vi "V(I)_K2636B_PK.vi"() -> ()   [LabVIEW 2016]
uses:
  Application/Labview Drivers/Keithley 2600 Series/Public/Configure/Source/Configure Source (Limit).vi
  Application/Labview Drivers/Keithley 2600 Series/Public/Configure/Source/Configure Source (Range).vi
  Labview Drivers/Keithley 2600 Series/Public/Data/Read Measurement (Current and Voltage).vi
  Application/Labview Drivers/Keithley 2600 Series/Keithley 2600 Series.lvlib
panel:
  in  "4-point sense":bool=TRUE
  out "Resistance (ohm)":dbl=6608698.625453053 format="%#_13g"
  out "R vs V":cluster{dbl, "Field Reading":dbl}[](graph)=[{3.33548e-05, "Field Reading"=75621777.7515791}, {3.15428e-05, "Field Reading"=1576.9586497552782}, {3.19242e-05, "Field Reading"=797.9912862417107}, {3.13759e-05, "Field Reading"=522.8758932380546}, {3.35217e-05, "Field Reading"=418.980923086153}, {3.21865e-05, "Field Reading"=321.8392528597712}, {3.17812e-05, "Field Reading"=264.76169847630314}, {3.32117e-05, "Field Reading"=237.178992772874}, {3.36409e-05, "Field Reading"=210.20570114597783}, {3.27587e-05, "Field Reading"=181.93819631888212}, {3.33786e-05, "Field Reading"=166.85295529073022}, {3.28064e-05, "Field Reading"=149.08205184134948}, {3.19719e-05, "Field Reading"=133.19072177832584}, {3.27826e-05, "Field Reading"=126.06025648420527}, {3.20911e-05, "Field Reading"=114.59142718391132}, {3.31402e-05, "Field Reading"=110.44487620850427}, {3.37124e-05, "Field Reading"=105.33413320335445}, {3.19719e-05, "Field Reading"=94.01619676064786}, {3.04937e-05, "Field Reading"=84.68449203801315}, {3.25918e-05, "Field Reading"=85.75074458792453}, {3.10421e-05, "Field Reading"=77.58915025132285}, {3.25918e-05, "Field Reading"=77.58529983788686}, {3.25441e-05, "Field Reading"=73.94974595758991}, {3.20196e-05, "Field Reading"=69.59678138034617}, {3.03268e-05, "Field Reading"=63.16977862207446}, {3.09229e-05, "Field Reading"=61.83293874874027}, {2.90155e-05, "Field Reading"=55.7893826068565}, {3.00884e-05, "Field Reading"=55.70935537385946}, {2.91348e-05, "Field Reading"=52.01797565038539}, {3.13044e-05, "Field Reading"=53.963613295592836}, {3.03507e-05, "Field Reading"=50.576660617604276}, {3.16858e-05, "Field Reading"=51.09747542754856}, {2.99692e-05, "Field Reading"=46.81992516735797}, {3.11136e-05, "Field Reading"=47.133891118311915}, {2.86102e-05, "Field Reading"=42.06646189857952}, {2.87533e-05, "Field Reading"=41.0698650349161}, {2.96354e-05, "Field Reading"=41.153761765498245}, {2.9397e-05, "Field Reading"=39.719717718017975}, {2.84672e-05, "Field Reading"=37.45112588078662}, {3.11852e-05, "Field Reading"=39.97569554828587}, {3.11375e-05, "Field Reading"=38.91623214633878}, {3.05891e-05, "Field Reading"=37.29918631973379}, {2.89917e-05, "Field Reading"=34.50932732778487}, {2.94447e-05, "Field Reading"=34.2332067232401}, {2.97546e-05, "Field Reading"=33.807857890329494}, {3.3474e-05, "Field Reading"=37.18854014371481}, {3.24249e-05, "Field Reading"=35.240319614653934}, {3.03745e-05, "Field Reading"=32.30941386833285}, {3.14236e-05, "Field Reading"=32.72933689544373}, {3.10183e-05, "Field Reading"=31.647871099788087}, {3.16858e-05, "Field Reading"=31.682314945356012}, {3.33786e-05, "Field Reading"=32.719947457676966}, {3.29733e-05, "Field Reading"=31.702352681017988}, {3.20911e-05, "Field Reading"=30.27290908061808}, {3.47137e-05, "Field Reading"=32.141124402799896}, {3.34263e-05, "Field Reading"=30.38284992319369}, {3.31163e-05, "Field Reading"=29.563901585487788}, {3.33548e-05, "Field Reading"=29.25526036504609}, {3.34263e-05, "Field Reading"=28.813043590693987}, {2.95877e-05, "Field Reading"=25.07283466235054}, {3.04461e-05, "Field Reading"=25.370904303189892}, {3.06368e-05, "Field Reading"=25.108220850851097}, {3.06606e-05, "Field Reading"=24.723299600854734}, {3.10898e-05, "Field Reading"=24.672290514320178}, {3.18766e-05, "Field Reading"=24.901259256944662}, {3.20196e-05, "Field Reading"=24.628756470705873}, {3.20911e-05, "Field Reading"=24.307204047779553}, {3.09706e-05, "Field Reading"=23.108938964333678}, {3.23057e-05, "Field Reading"=23.751396894482998}, {3.05414e-05, "Field Reading"=22.1292042836234}, {3.20196e-05, "Field Reading"=22.869509320762806}, {3.19719e-05, "Field Reading"=22.514471219525934}, {3.25918e-05, "Field Reading"=22.630051381752537}, {3.37362e-05, "Field Reading"=23.103979619090666}, {3.12805e-05, "Field Reading"=21.133188303967138}, {3.00407e-05, "Field Reading"=20.025531290830067}, {2.97308e-05, "Field Reading"=19.558450101966976}, {3.01838e-05, "Field Reading"=19.596816080610814}, {3.09944e-05, "Field Reading"=19.865658248942445}, {3.03745e-05, "Field Reading"=19.222298866577646}, {3.02315e-05, "Field Reading"=18.892916289097897}, {3.01838e-05, "Field Reading"=18.63048027010178}, {3.02315e-05, "Field Reading"=18.43282990567591}, {3.21388e-05, "Field Reading"=19.358273953295065}, {3.12805e-05, "Field Reading"=18.617239716936776}, {2.99454e-05, "Field Reading"=17.613179858484738}, {3.31879e-05, "Field Reading"=19.293608115571317}, {3.3021e-05, "Field Reading"=18.976168447184982}, {3.1352e-05, "Field Reading"=17.81090400904407}, {3.12805e-05, "Field Reading"=17.571044190919153}, {3.20435e-05, "Field Reading"=17.79967004216128}, {3.23057e-05, "Field Reading"=17.748531746685785}, {3.35693e-05, "Field Reading"=18.242499334300632}, {3.11613e-05, "Field Reading"=16.752036126118863}, {3.07322e-05, "Field Reading"=16.344393683953005}, {3.22819e-05, "Field Reading"=16.988148990138193}, {3.32356e-05, "Field Reading"=17.308134962999222}, {3.12805e-05, "Field Reading"=16.122306978661992}, {3.08514e-05, "Field Reading"=15.738904193449649}, {3.02553e-05, "Field Reading"=15.277831079511598}, {2.97546e-05, "Field Reading"=14.87499437587174}, {3.06845e-05, "Field Reading"=15.188391593161276}, {3.32356e-05, "Field Reading"=16.290124152669062}, {3.25203e-05, "Field Reading"=15.785020871760022}, {3.14951e-05, "Field Reading"=15.140637544046882}, {3.14236e-05, "Field Reading"=14.96162416439713}, {3.09467e-05, "Field Reading"=14.595847639889824}, {3.08752e-05, "Field Reading"=14.425978273566171}, {2.91109e-05, "Field Reading"=13.47589597355825}, {3.0756e-05, "Field Reading"=14.106962663975784}, {3.11613e-05, "Field Reading"=14.162038594035467}, {3.13282e-05, "Field Reading"=14.109767961374938}, {3.24011e-05, "Field Reading"=14.46277524092648}, {3.09706e-05, "Field Reading"=13.702228947112278}, {3.32594e-05, "Field Reading"=14.585984747152699}, {3.12567e-05, "Field Reading"=13.588569788976706}, {3.10898e-05, "Field Reading"=13.398696753951974}, {3.07798e-05, "Field Reading"=13.151849731235632}, {3.32117e-05, "Field Reading"=14.07096555522603}, {3.18289e-05, "Field Reading"=13.371970406718567}, {3.18289e-05, "Field Reading"=13.260605101114049}, {3.46661e-05, "Field Reading"=14.322526534979898}, {3.24726e-05, "Field Reading"=13.306588426202905}, {3.2711e-05, "Field Reading"=13.295479025000915}, {3.23772e-05, "Field Reading"=13.053796128678501}, {3.49998e-05, "Field Reading"=13.998408171917434}, {3.3164e-05, "Field Reading"=13.159064216106405}, {3.22104e-05, "Field Reading"=12.679462753310554}, {3.3164e-05, "Field Reading"=12.953017775052437}, {3.53336e-05, "Field Reading"=13.693548449604894}, {3.56197e-05, "Field Reading"=13.698462082783712}, {3.41654e-05, "Field Reading"=13.039084355190194}, {3.438e-05, "Field Reading"=13.020754431146795}, {3.28064e-05, "Field Reading"=12.331564149212888}, {3.47137e-05, "Field Reading"=12.951230067827217}, {3.28302e-05, "Field Reading"=12.158027471123473}, {5.20706e-05, "Field Reading"=19.141773212854652}, {5.3215e-05, "Field Reading"=19.41997357876375}, {5.37634e-05, "Field Reading"=19.47695228158646}, {5.20945e-05, "Field Reading"=18.736804623911553}, {5.32627e-05, "Field Reading"=19.020287039649183}, {5.1713e-05, "Field Reading"=18.33599262489806}, {5.22375e-05, "Field Reading"=18.391672651992057}, {5.36203e-05, "Field Reading"=18.745734862257024}, {5.35727e-05, "Field Reading"=18.599242458434162}, {5.24282e-05, "Field Reading"=18.076508007654247}, {5.28336e-05, "Field Reading"=18.091654025401237}, {5.27859e-05, "Field Reading"=17.952616918739306}, {5.31435e-05, "Field Reading"=17.952308243194853}, {5.19037e-05, "Field Reading"=17.41489454506412}, {5.29528e-05, "Field Reading"=17.648697831607997}, {5.46932e-05, "Field Reading"=18.10817253572422}, {5.49078e-05, "Field Reading"=18.059815875250386}, {5.23329e-05, "Field Reading"=17.100634253616487}, {5.56707e-05, "Field Reading"=18.072262169488226}, {5.28812e-05, "Field Reading"=17.056140780926455}, {5.53131e-05, "Field Reading"=17.726341899570244}, {5.43594e-05, "Field Reading"=17.30987112983502}, {5.45979e-05, "Field Reading"=17.27590298542883}, {5.47171e-05, "Field Reading"=17.2049039090406}, {5.50985e-05, "Field Reading"=17.215806477818816}, {5.63622e-05, "Field Reading"=17.50139732458919}, {5.61714e-05, "Field Reading"=17.334658268552435}, {5.70059e-05, "Field Reading"=17.484434329740704}, {5.66244e-05, "Field Reading"=17.261694636243085}, {5.7292e-05, "Field Reading"=17.358687221252666}, {5.6839e-05, "Field Reading"=17.117808978274095}, {5.6076e-05, "Field Reading"=16.78701009447857}, {5.76735e-05, "Field Reading"=17.162688965599333}, {5.94378e-05, "Field Reading"=17.583223138295512}, {5.65767e-05, "Field Reading"=16.638493096298912}, {5.73397e-05, "Field Reading"=16.76364136027692}, {5.84126e-05, "Field Reading"=16.978185993111367}, {5.8651e-05, "Field Reading"=16.949098664323984}, {5.5933e-05, "Field Reading"=16.07099245195195}, {5.68867e-05, "Field Reading"=16.251578400059422}, {5.94139e-05, "Field Reading"=16.87650368838606}, {5.85318e-05, "Field Reading"=16.532118435583776}, {5.99623e-05, "Field Reading"=16.84121389150248}, {6.00338e-05, "Field Reading"=16.76720393919166}, {6.00576e-05, "Field Reading"=16.680813242973002}, {6.03437e-05, "Field Reading"=16.66782676908714}, {6.06775e-05, "Field Reading"=16.667353385523967}, {5.86271e-05, "Field Reading"=16.01627659836032}, {6.02484e-05, "Field Reading"=16.369757123410867}, {6.00576e-05, "Field Reading"=16.229853747121965}, {6.08444e-05, "Field Reading"=16.354175066255962}, {6.02961e-05, "Field Reading"=16.119581344989374}, {6.001e-05, "Field Reading"=15.957899439439228}, {6.31094e-05, "Field Reading"=16.69344450058061}, {6.26802e-05, "Field Reading"=16.49274958097288}, {6.08444e-05, "Field Reading"=15.925935620317974}, {6.19412e-05, "Field Reading"=16.12867275624668}, {6.21319e-05, "Field Reading"=16.09392889151371}, {6.39439e-05, "Field Reading"=16.47809325506244}, {6.33001e-05, "Field Reading"=16.228631054320964}, {6.20842e-05, "Field Reading"=15.835867036689383}, {6.41823e-05, "Field Reading"=16.28810488168834}, {6.37531e-05, "Field Reading"=16.096910048528247}, {6.51598e-05, "Field Reading"=16.369546921907776}, {6.55174e-05, "Field Reading"=16.37718002364687}, {6.50883e-05, "Field Reading"=16.188985034311397}, {6.44922e-05, "Field Reading"=15.961479919514714}, {6.49452e-05, "Field Reading"=15.994581881318572}, {6.64234e-05, "Field Reading"=16.277931078425127}, {6.43253e-05, "Field Reading"=15.687069720255673}, {6.5732e-05, "Field Reading"=15.95247167205842}, {6.71148e-05, "Field Reading"=16.209503291904763}, {6.58512e-05, "Field Reading"=15.82794127544202}, {6.46591e-05, "Field Reading"=15.466464143902789}, {6.61135e-05, "Field Reading"=15.739173493121173}, {6.44922e-05, "Field Reading"=15.280556516464719}, {6.61612e-05, "Field Reading"=15.602216719726448}, {6.61135e-05, "Field Reading"=15.517888871415597}, {6.53028e-05, "Field Reading"=15.256095167786489}, {6.53744e-05, "Field Reading"=15.201298429514159}, {6.59227e-05, "Field Reading"=15.258012327191341}, {6.62088e-05, "Field Reading"=15.253726529201705}, {6.58035e-05, "Field Reading"=15.090849881550009}, {6.51598e-05, "Field Reading"=14.875138399022934}, {6.6185e-05, "Field Reading"=15.040028723421178}, {6.44922e-05, "Field Reading"=14.589180079401885}, {6.62088e-05, "Field Reading"=14.910112081215532}, {6.67334e-05, "Field Reading"=14.960901419565433}, {6.73532e-05, "Field Reading"=15.032518692110257}, {6.75201e-05, "Field Reading"=15.002933033512129}, {6.7687e-05, "Field Reading"=14.972979310314317}, {6.74486e-05, "Field Reading"=14.85458938155614}, {6.63996e-05, "Field Reading"=14.559559702228897}, {6.4683e-05, "Field Reading"=14.12129164092365}, {6.57082e-05, "Field Reading"=14.282807775659656}, {6.5732e-05, "Field Reading"=14.225734963121992}, {6.73771e-05, "Field Reading"=14.519080547947565}, {6.92368e-05, "Field Reading"=14.855929021252857}, {6.73771e-05, "Field Reading"=14.395247526444766}, {6.82592e-05, "Field Reading"=14.521689182001914}, {6.88076e-05, "Field Reading"=14.575935839072327}, {6.62565e-05, "Field Reading"=13.97642487538471}, {6.82831e-05, "Field Reading"=14.343501604853211}, {6.65903e-05, "Field Reading"=13.929509760444471}, {6.88076e-05, "Field Reading"=14.333423601708155}, {6.85453e-05, "Field Reading"=14.21965953456724}, {6.48737e-05, "Field Reading"=13.401995620377638}, {6.90699e-05, "Field Reading"=14.210188475061669}, {7.12872e-05, "Field Reading"=14.606356647597815}, {6.96421e-05, "Field Reading"=14.21113634647681}, {7.20501e-05, "Field Reading"=14.64284117467737}, {7.27654e-05, "Field Reading"=14.727959794601093}, {7.08103e-05, "Field Reading"=14.27454340200782}, {7.32422e-05, "Field Reading"=14.705585906833958}, {7.10487e-05, "Field Reading"=14.208233927203715}, {7.09057e-05, "Field Reading"=14.179608602270953}, {7.0262e-05, "Field Reading"=14.107220659482751}, {7.00235e-05, "Field Reading"=14.11596201258318}, {7.04288e-05, "Field Reading"=14.25499530425208}, {7.01189e-05, "Field Reading"=14.250331774551826}, {7.08103e-05, "Field Reading"=14.449489239961311}, {6.99759e-05, "Field Reading"=14.337707840304883}, {7.02143e-05, "Field Reading"=14.445633143301533}, {7.15733e-05, "Field Reading"=14.786069466738558}, {7.06196e-05, "Field Reading"=14.65000155587134}, {7.11679e-05, "Field Reading"=14.825101551921675}, {6.81162e-05, "Field Reading"=14.248700978136268}, {6.71864e-05, "Field Reading"=14.113159193790635}, {6.73532e-05, "Field Reading"=14.207797358129174}, {6.7234e-05, "Field Reading"=14.242711186525412}, {6.69956e-05, "Field Reading"=14.252957682955111}, {6.69718e-05, "Field Reading"=14.308715540466917}, {6.87599e-05, "Field Reading"=14.753697012350553}, {6.73294e-05, "Field Reading"=14.50889547813195}, {6.65903e-05, "Field Reading"=14.41164440039043}, {6.28948e-05, "Field Reading"=13.67144518471019}, {6.51121e-05, "Field Reading"=14.21512592566718}, {6.77824e-05, "Field Reading"=14.86289910558249}, {6.72102e-05, "Field Reading"=14.802215590622282}, {6.58989e-05, "Field Reading"=14.577532086590658}, {6.60658e-05, "Field Reading"=14.679853525433067}, {6.79493e-05, "Field Reading"=15.165629575402637}, {6.61612e-05, "Field Reading"=14.832686918506896}, {6.77347e-05, "Field Reading"=15.25377658472431}, {6.49214e-05, "Field Reading"=14.686338515969805}, {6.53744e-05, "Field Reading"=14.85589366832024}, {6.54936e-05, "Field Reading"=14.951374747742237}, {6.3777e-05, "Field Reading"=14.62620916141875}, {6.48737e-05, "Field Reading"=14.946238540987496}, {6.44922e-05, "Field Reading"=14.9270568847515}, {6.34193e-05, "Field Reading"=14.746856782768637}, {6.45399e-05, "Field Reading"=15.078006728343146}, {6.3014e-05, "Field Reading"=14.79056055506265}, {6.42538e-05, "Field Reading"=15.15262567092094}, {6.6185e-05, "Field Reading"=15.681865569793011}, {6.60658e-05, "Field Reading"=15.728005104129963}, {6.51598e-05, "Field Reading"=15.586455338305578}, {6.46353e-05, "Field Reading"=15.535800558118071}, {6.57082e-05, "Field Reading"=15.869897571025232}, {6.36101e-05, "Field Reading"=15.43762104231081}, {6.30617e-05, "Field Reading"=15.379064453272658}, {6.22272e-05, "Field Reading"=15.249821101232197}, {6.17981e-05, "Field Reading"=15.21974490135184}, {6.36339e-05, "Field Reading"=15.749289060817786}, {6.23465e-05, "Field Reading"=15.507266563361993}, {6.19888e-05, "Field Reading"=15.495340559132904}, {6.07967e-05, "Field Reading"=15.273633965582212}, {6.16312e-05, "Field Reading"=15.56131234629621}, {6.22749e-05, "Field Reading"=15.804207694650287}, {6.32763e-05, "Field Reading"=16.140101621246597}, {6.21557e-05, "Field Reading"=15.935356839781667}, {6.32048e-05, "Field Reading"=16.287714017708968}, {6.53744e-05, "Field Reading"=16.933960187019984}, {6.43969e-05, "Field Reading"=16.76823568316924}, {6.08206e-05, "Field Reading"=15.919872684155147}, {6.02484e-05, "Field Reading"=15.853006493984907}, {6.33001e-05, "Field Reading"=16.74393198747249}, {6.1655e-05, "Field Reading"=16.39542614014094}, {6.02484e-05, "Field Reading"=16.106958390811972}, {6.1655e-05, "Field Reading"=16.572187324447167}, {6.13689e-05, "Field Reading"=16.584306646272584}, {5.96762e-05, "Field Reading"=16.214420014998208}, {6.10828e-05, "Field Reading"=16.687192320090915}, {6.04391e-05, "Field Reading"=16.601913478680068}, {6.29902e-05, "Field Reading"=17.398925518250998}, {6.03914e-05, "Field Reading"=16.773571751949095}, {5.93424e-05, "Field Reading"=16.57414493271739}, {6.05345e-05, "Field Reading"=17.00192391411198}, {5.87702e-05, "Field Reading"=16.599453747927548}, {5.83649e-05, "Field Reading"=16.57848840512197}, {6.07014e-05, "Field Reading"=17.341374365068937}, {5.79834e-05, "Field Reading"=16.660173085542876}, {6.0606e-05, "Field Reading"=17.51410959972951}, {5.97239e-05, "Field Reading"=17.359327994884392}, {5.9557e-05, "Field Reading"=17.41193461717249}, {5.98431e-05, "Field Reading"=17.59915184952093}, {5.81503e-05, "Field Reading"=17.202449450500687}, {5.89848e-05, "Field Reading"=17.552910367813354}, {5.88655e-05, "Field Reading"=17.62218523419211}, {5.87702e-05, "Field Reading"=17.699415141275608}, {5.79834e-05, "Field Reading"=17.56822513157217}, {5.3525e-05, "Field Reading"=16.316906174359975}, {5.47409e-05, "Field Reading"=16.7897815278634}, {5.61237e-05, "Field Reading"=17.31993790909175}, {5.73635e-05, "Field Reading"=17.812372881882233}, {5.7888e-05, "Field Reading"=18.087399936259164}, {5.66244e-05, "Field Reading"=17.804623434119836}, {5.72443e-05, "Field Reading"=18.11327859256095}, {5.68151e-05, "Field Reading"=18.091906660382882}, {5.86271e-05, "Field Reading"=18.788388630908315}, {5.83887e-05, "Field Reading"=18.832573756374156}, {5.54085e-05, "Field Reading"=17.98720312682604}, {5.68628e-05, "Field Reading"=18.58079273273862}, {5.68151e-05, "Field Reading"=18.687087628357354}, {5.65052e-05, "Field Reading"=18.708162961246217}, {5.56231e-05, "Field Reading"=18.538623312302736}, {5.50032e-05, "Field Reading"=18.454786725405395}, {5.42879e-05, "Field Reading"=18.338895907791883}, {5.49793e-05, "Field Reading"=18.698597757364066}, {5.19753e-05, "Field Reading"=17.79787077399317}, {5.30243e-05, "Field Reading"=18.28209796092872}, {5.31197e-05, "Field Reading"=18.442099050462616}, {5.33104e-05, "Field Reading"=18.637523685664142}, {5.48124e-05, "Field Reading"=19.298306146950814}, {5.23329e-05, "Field Reading"=18.555791937027976}, {5.50509e-05, "Field Reading"=19.658929400421382}, {5.13792e-05, "Field Reading"=18.479533005074938}, {5.10931e-05, "Field Reading"=18.50951140607962}, {5.09977e-05, "Field Reading"=18.610669138469625}, {5.0211e-05, "Field Reading"=18.458162087447523}, {5.12838e-05, "Field Reading"=18.99203045610085}, {5.13792e-05, "Field Reading"=19.169054441260744}, {5.25713e-05, "Field Reading"=19.76112075900073}, {5.08785e-05, "Field Reading"=19.26938546724335}, {5.095e-05, "Field Reading"=19.445006316287625}, {5.03063e-05, "Field Reading"=19.34671666185944}, {4.94957e-05, "Field Reading"=19.1822237035372}, {5.04017e-05, "Field Reading"=19.68578023754936}, {4.99964e-05, "Field Reading"=19.680910110811503}, {4.89235e-05, "Field Reading"=19.412469595787652}, {5.04017e-05, "Field Reading"=20.15874476050299}, {5.10216e-05, "Field Reading"=20.57115210160266}, {5.28336e-05, "Field Reading"=21.474803476055374}, {5.06401e-05, "Field Reading"=20.751672956902667}, {4.96149e-05, "Field Reading"=20.49931414027897}, {4.9758e-05, "Field Reading"=20.730945179111565}, {4.8399e-05, "Field Reading"=20.333920116292262}, {4.91858e-05, "Field Reading"=20.839498012897103}, {4.92811e-05, "Field Reading"=21.057959372035583}, {5.00441e-05, "Field Reading"=21.568036754026433}, {5.03302e-05, "Field Reading"=21.88117348358375}, {4.67062e-05, "Field Reading"=20.483558315571575}, {4.73261e-05, "Field Reading"=20.938899212459074}, {4.62055e-05, "Field Reading"=20.625153442696128}, {4.76599e-05, "Field Reading"=21.4657160358153}, {4.59194e-05, "Field Reading"=20.86951384123146}, {4.51803e-05, "Field Reading"=20.723387274328488}, {4.64678e-05, "Field Reading"=21.510978200991584}, {4.673e-05, "Field Reading"=21.834203960340528}, {4.52995e-05, "Field Reading"=21.365370738080305}, {4.673e-05, "Field Reading"=22.249626236751638}, {4.49896e-05, "Field Reading"=21.62795169602338}, {4.52757e-05, "Field Reading"=21.976574862390663}, {4.60148e-05, "Field Reading"=22.55406332712479}, {4.68969e-05, "Field Reading"=23.213758897545816}, {4.84943e-05, "Field Reading"=24.243998280223572}, {4.60863e-05, "Field Reading"=23.27250049235213}, {4.55618e-05, "Field Reading"=23.24380028262855}, {4.59909e-05, "Field Reading"=23.704205751984333}, {4.56095e-05, "Field Reading"=23.752102612707855}, {3.34024e-05, "Field Reading"=17.577712640835248}, {3.438e-05, "Field Reading"=18.284413574501805}, {3.49998e-05, "Field Reading"=18.815579388758973}, {3.31879e-05, "Field Reading"=18.0351378669478}, {3.29494e-05, "Field Reading"=18.10197724438389}, {3.37124e-05, "Field Reading"=18.726510206915705}, {3.44992e-05, "Field Reading"=19.378742430880884}, {3.40462e-05, "Field Reading"=19.34135478446611}, {3.38316e-05, "Field Reading"=19.441772261011984}, {3.53336e-05, "Field Reading"=20.54064109569929}, {3.1209e-05, "Field Reading"=18.356075755793434}, {3.32594e-05, "Field Reading"=19.79455193634205}, {3.05176e-05, "Field Reading"=18.38132811323596}, {3.03984e-05, "Field Reading"=18.53436659736237}, {3.16143e-05, "Field Reading"=19.51331366425124}, {3.10659e-05, "Field Reading"=19.41424607539246}, {3.24965e-05, "Field Reading"=20.564801923807117}, {3.15666e-05, "Field Reading"=20.23227642432749}, {3.24488e-05, "Field Reading"=21.06722934588541}, {3.19719e-05, "Field Reading"=21.032622639151114}, {3.26633e-05, "Field Reading"=21.77364628398872}, {3.19958e-05, "Field Reading"=21.616446870608584}, {3.34263e-05, "Field Reading"=22.89159019312423}, {3.2258e-05, "Field Reading"=22.398122496024886}, {3.29494e-05, "Field Reading"=23.202659023850938}, {3.09467e-05, "Field Reading"=22.103206913791873}, {3.32117e-05, "Field Reading"=24.064182359632788}, {3.47137e-05, "Field Reading"=25.521776849782377}, {3.54528e-05, "Field Reading"=26.45356255456316}, {3.25203e-05, "Field Reading"=24.63229891761284}, {3.37124e-05, "Field Reading"=25.93101962956126}, {3.00646e-05, "Field Reading"=23.48595042613525}, {3.00884e-05, "Field Reading"=23.877597987477284}, {3.34024e-05, "Field Reading"=26.934378376634893}, {3.08275e-05, "Field Reading"=25.26471504204298}, {3.39746e-05, "Field Reading"=28.31122295923469}, {3.14474e-05, "Field Reading"=26.64875812451804}, {3.22819e-05, "Field Reading"=27.82706514149764}, {3.22819e-05, "Field Reading"=28.313978985036925}, {3.08514e-05, "Field Reading"=27.541958291672618}, {3.20435e-05, "Field Reading"=29.125953261768633}, {3.16858e-05, "Field Reading"=29.338160404436955}, {3.16858e-05, "Field Reading"=29.89057223176047}, {3.31163e-05, "Field Reading"=31.839840783009166}, {3.18766e-05, "Field Reading"=31.246973484291523}, {3.08514e-05, "Field Reading"=30.847698276206852}, {3.22342e-05, "Field Reading"=32.88804726772973}, {3.33548e-05, "Field Reading"=34.74042172031476}, {3.13759e-05, "Field Reading"=33.37417896556309}, {3.25918e-05, "Field Reading"=35.42136489163878}, {3.07798e-05, "Field Reading"=34.19483852332441}, {3.3474e-05, "Field Reading"=38.03332034272482}, {3.31402e-05, "Field Reading"=38.529292083754775}, {3.25441e-05, "Field Reading"=38.73735005154013}, {3.39746e-05, "Field Reading"=41.426679705504355}, {3.42607e-05, "Field Reading"=42.819023956167015}, {3.19719e-05, "Field Reading"=40.98352039953033}, {3.1352e-05, "Field Reading"=41.24563067584581}, {3.17335e-05, "Field Reading"=42.875691772233985}, {3.07798e-05, "Field Reading"=42.74164879967117}, {3.14951e-05, "Field Reading"=44.98458145689879}, {3.40462e-05, "Field Reading"=50.057487995153956}, {3.27826e-05, "Field Reading"=49.660899612045526}, {3.39985e-05, "Field Reading"=53.112614646293444}, {3.46422e-05, "Field Reading"=55.86298312606429}, {3.2568e-05, "Field Reading"=54.26959832698733}, {3.45469e-05, "Field Reading"=59.550478515086326}, {3.15905e-05, "Field Reading"=56.40012568869909}, {3.15666e-05, "Field Reading"=58.443462773225306}, {3.2115e-05, "Field Reading"=61.746553613658655}, {3.16381e-05, "Field Reading"=63.26114384776423}, {3.10898e-05, "Field Reading"=64.75571172379605}, {3.14951e-05, "Field Reading"=68.45287644615615}, {3.11613e-05, "Field Reading"=70.80440077799794}, {3.31163e-05, "Field Reading"=78.82937674511606}, {3.14951e-05, "Field Reading"=78.71748024883593}, {3.2711e-05, "Field Reading"=86.06142245631945}, {3.16858e-05, "Field Reading"=87.99142462809046}, {3.21388e-05, "Field Reading"=94.50170103532331}, {3.12328e-05, "Field Reading"=97.58023950786226}, {2.98738e-05, "Field Reading"=99.55046369886065}, {3.09944e-05, "Field Reading"=110.66543365479714}, {2.94447e-05, "Field Reading"=113.2153170022724}, {2.99931e-05, "Field Reading"=124.93481068021826}, {3.13997e-05, "Field Reading"=142.6759725005339}, {3.26395e-05, "Field Reading"=163.14366259134485}, {3.34263e-05, "Field Reading"=185.62844655719135}, {3.40939e-05, "Field Reading"=213.00433581986982}, {3.02553e-05, "Field Reading"=216.03213138164944}, {3.1805e-05, "Field Reading"=264.9158316466345}, {3.27349e-05, "Field Reading"=327.322814174866}, {3.21627e-05, "Field Reading"=401.99355064493557}, {3.35932e-05, "Field Reading"=559.8241529695852}, {3.37124e-05, "Field Reading"=842.6857038586808}, {3.30925e-05, "Field Reading"=1654.409926709528}, {3.36409e-05, "Field Reading"=44793673.662051156}, {3.30687e-05, "Field Reading"=-1653.6913221549337}, {3.56913e-05, "Field Reading"=-892.3025768079782}, {3.51429e-05, "Field Reading"=-585.7081667380546}, {3.39746e-05, "Field Reading"=-424.67719153510575}, {3.44992e-05, "Field Reading"=-344.9975199603194}, {3.33309e-05, "Field Reading"=-277.87559712877976}, {3.34978e-05, "Field Reading"=-239.36745675024835}, {3.21627e-05, "Field Reading"=-201.08977004164012}, {3.438e-05, "Field Reading"=-191.04670030451888}, {3.39031e-05, "Field Reading"=-169.5502578028496}, {3.50475e-05, "Field Reading"=-159.32709617587693}, {3.47137e-05, "Field Reading"=-144.65910180064924}, {3.48568e-05, "Field Reading"=-134.0842123079527}, {3.56197e-05, "Field Reading"=-127.22502803831784}, {3.52859e-05, "Field Reading"=-117.63260625335455}, {3.50475e-05, "Field Reading"=-109.53781433813188}, {3.65019e-05, "Field Reading"=-107.36768724391196}, {3.41654e-05, "Field Reading"=-94.91127087662375}, {3.38554e-05, "Field Reading"=-89.09761277537561}, {3.38316e-05, "Field Reading"=-84.58344063063312}, {3.44276e-05, "Field Reading"=-81.97555086743465}, {3.51906e-05, "Field Reading"=-79.98081765866343}, {3.57866e-05, "Field Reading"=-77.80000086959924}, {3.44992e-05, "Field Reading"=-71.87707693109017}, {3.51667e-05, "Field Reading"=-70.33536939034293}, {3.61443e-05, "Field Reading"=-69.51080904879217}, {3.47376e-05, "Field Reading"=-64.32984192358404}, {3.52383e-05, "Field Reading"=-62.927108892008015}, {3.44753e-05, "Field Reading"=-59.441504723381726}, {3.36885e-05, "Field Reading"=-56.147312842290525}, {3.56436e-05, "Field Reading"=-57.490048322892406}, {3.74079e-05, "Field Reading"=-58.45103103656793}, {3.49522e-05, "Field Reading"=-52.95771830994452}, {3.49045e-05, "Field Reading"=-51.33052448915065}, {3.48091e-05, "Field Reading"=-49.728493406268434}, {3.5882e-05, "Field Reading"=-49.836318762439284}, {3.52621e-05, "Field Reading"=-47.65200164326101}, {3.55959e-05, "Field Reading"=-46.83671052631579}, {3.7384e-05, "Field Reading"=-47.92894249655123}, {3.42846e-05, "Field Reading"=-42.85671427607121}, {3.64065e-05, "Field Reading"=-44.39865803405159}, {3.438e-05, "Field Reading"=-40.9293023089698}, {3.54528e-05, "Field Reading"=-41.225336521019194}, {3.54052e-05, "Field Reading"=-40.23363901862521}, {3.77178e-05, "Field Reading"=-41.90936515608593}, {3.50237e-05, "Field Reading"=-38.06973569220468}, {3.33786e-05, "Field Reading"=-35.50975335750396}, {3.56913e-05, "Field Reading"=-37.179444443287004}, {3.55482e-05, "Field Reading"=-36.2743397327706}, {3.39985e-05, "Field Reading"=-33.99945198465557}, {3.51906e-05, "Field Reading"=-34.501264730680994}, {3.37362e-05, "Field Reading"=-32.44021347180152}, {3.35932e-05, "Field Reading"=-31.69409012000906}, {3.38316e-05, "Field Reading"=-31.32874644639732}, {3.48091e-05, "Field Reading"=-31.648664375465966}, {3.63112e-05, "Field Reading"=-32.42505692726704}, {3.67641e-05, "Field Reading"=-32.248927640985606}, {3.53813e-05, "Field Reading"=-30.50164658011345}, {3.28779e-05, "Field Reading"=-27.86357164649649}, {3.55244e-05, "Field Reading"=-29.605146924012868}, {3.31163e-05, "Field Reading"=-27.146288281198764}, {3.23296e-05, "Field Reading"=-26.074781430461012}, {3.39746e-05, "Field Reading"=-26.966964583366405}, {3.29971e-05, "Field Reading"=-25.778782978257983}, {3.39508e-05, "Field Reading"=-26.116401790796782}, {3.35217e-05, "Field Reading"=-25.39580445010114}, {3.19242e-05, "Field Reading"=-23.824918840255236}, {3.36885e-05, "Field Reading"=-24.772413083122537}, {3.35932e-05, "Field Reading"=-24.34501550859495}, {3.17097e-05, "Field Reading"=-22.649623931257633}, {3.22104e-05, "Field Reading"=-22.6836997704193}, {3.02315e-05, "Field Reading"=-20.994534608359896}, {3.11852e-05, "Field Reading"=-21.360164934895923}, {2.92301e-05, "Field Reading"=-19.75100173656862}, {3.04937e-05, "Field Reading"=-20.330488699246615}, {3.19481e-05, "Field Reading"=-21.017933738585825}, {3.29494e-05, "Field Reading"=-21.3958532198261}, {3.30448e-05, "Field Reading"=-21.182971467400016}, {3.14713e-05, "Field Reading"=-19.919174657425867}, {3.20911e-05, "Field Reading"=-20.057940397019852}, {3.2115e-05, "Field Reading"=-19.824930706882398}, {3.00646e-05, "Field Reading"=-18.33319104823465}, {3.22342e-05, "Field Reading"=-19.417841846231692}, {3.2568e-05, "Field Reading"=-19.385714285714283}, {3.14713e-05, "Field Reading"=-18.512747208790692}, {3.28064e-05, "Field Reading"=-19.073931951905855}, {3.39985e-05, "Field Reading"=-19.540041610630254}, {3.46899e-05, "Field Reading"=-19.71106641210964}, {3.34024e-05, "Field Reading"=-18.764655322543494}, {2.76566e-05, "Field Reading"=-15.36409492911426}, {3.20911e-05, "Field Reading"=-17.63189125633221}, {3.29971e-05, "Field Reading"=-17.93330398534775}, {3.36885e-05, "Field Reading"=-18.112486290027743}, {3.25918e-05, "Field Reading"=-17.336617126078494}, {3.3474e-05, "Field Reading"=-17.617152961980548}, {3.34024e-05, "Field Reading"=-17.396449087793673}, {3.438e-05, "Field Reading"=-17.72128409723511}, {3.38078e-05, "Field Reading"=-17.248701543861795}, {3.35932e-05, "Field Reading"=-16.96634831489048}, {3.2711e-05, "Field Reading"=-16.35582711654233}, {3.15666e-05, "Field Reading"=-15.627493885957005}, {3.15189e-05, "Field Reading"=-15.449835300576447}, {3.27349e-05, "Field Reading"=-15.890265332077703}, {3.23534e-05, "Field Reading"=-15.55422011115171}, {3.40462e-05, "Field Reading"=-16.212476190476192}, {3.46899e-05, "Field Reading"=-16.363314748252343}, {3.5429e-05, "Field Reading"=-16.555839567844412}, {3.49998e-05, "Field Reading"=-16.202785969233048}, {3.52144e-05, "Field Reading"=-16.15280173204653}, {3.41892e-05, "Field Reading"=-15.54019226835754}, {3.50475e-05, "Field Reading"=-15.787019936757327}, {3.47853e-05, "Field Reading"=-15.529151785714285}, {3.33071e-05, "Field Reading"=-14.737850502440297}, {3.40462e-05, "Field Reading"=-14.931692491217605}, {3.47614e-05, "Field Reading"=-15.11286367667774}, {3.35455e-05, "Field Reading"=-14.458768663149547}, {3.55959e-05, "Field Reading"=-15.21172805476853}, {3.56674e-05, "Field Reading"=-15.113112968902938}, {3.48568e-05, "Field Reading"=-14.645591213519213}, {3.65496e-05, "Field Reading"=-15.229190364879562}, {3.55244e-05, "Field Reading"=-14.678836912371752}, {3.42131e-05, "Field Reading"=-14.02130258024327}, {3.30687e-05, "Field Reading"=-13.442287758378894}, {3.48091e-05, "Field Reading"=-14.035644442652364}, {3.16381e-05, "Field Reading"=-12.655138758889928}, {3.34024e-05, "Field Reading"=-13.254920634920634}, {3.47614e-05, "Field Reading"=-13.684782394740468}, {3.29018e-05, "Field Reading"=-12.851663203287345}, {3.51906e-05, "Field Reading"=-13.639344516449103}, {3.57389e-05, "Field Reading"=-13.745413567379213}, {3.43323e-05, "Field Reading"=-13.103731240744416}, {3.22104e-05, "Field Reading"=-12.200724231451039}, {3.15905e-05, "Field Reading"=-11.875324226180185}, {3.26633e-05, "Field Reading"=-12.187161864678712}, {3.21388e-05, "Field Reading"=-11.90268616696233}, {1.4472e-05, "Field Reading"=-5.320412192243639}, {1.52588e-05, "Field Reading"=-5.568803488987427}, {1.4925e-05, "Field Reading"=-5.407549917935675}, {1.44243e-05, "Field Reading"=-5.18857845835087}, {1.4329e-05, "Field Reading"=-5.117225862900201}, {1.49727e-05, "Field Reading"=-5.30918568161268}, {1.19925e-05, "Field Reading"=-4.222517983331749}, {1.02758e-05, "Field Reading"=-3.592798878364819}, {1.20401e-05, "Field Reading"=-4.1804886686781915}, {1.14918e-05, "Field Reading"=-3.9626213341149295}, {1.1301e-05, "Field Reading"=-3.869953667398354}, {1.15871e-05, "Field Reading"=-3.9409625974008304}, {1.33038e-05, "Field Reading"=-4.4942992753745585}, {1.1611e-05, "Field Reading"=-3.8961126117812857}, {9.91821e-06, "Field Reading"=-3.305926743174463}, {9.29832e-06, "Field Reading"=-3.078832348811952}, {9.91821e-06, "Field Reading"=-3.2623222585133362}, {1.05858e-05, "Field Reading"=-3.4591856741389453}, {1.06335e-05, "Field Reading"=-3.452233311040264}, {1.05143e-05, "Field Reading"=-3.3915565103511454}, {1.04189e-05, "Field Reading"=-3.3392732948517843}, {1.00613e-05, "Field Reading"=-3.204143830272381}, {1.01328e-05, "Field Reading"=-3.2064909543715525}, {9.2268e-06, "Field Reading"=-2.90130871449145}, {9.72748e-06, "Field Reading"=-3.039657020364416}, {8.7738e-06, "Field Reading"=-2.724647222498261}, {1.0705e-05, "Field Reading"=-3.303879782601315}, {9.82285e-06, "Field Reading"=-3.0130702314053646}, {1.10865e-05, "Field Reading"=-3.379978963735309}, {8.39233e-06, "Field Reading"=-2.5429761832616204}, {9.13143e-06, "Field Reading"=-2.7502650442744416}, {8.41618e-06, "Field Reading"=-2.5196936673692276}, {1.01805e-05, "Field Reading"=-3.0297844732659946}, {9.41753e-06, "Field Reading"=-2.78616904825301}, {7.77245e-06, "Field Reading"=-2.285960918566622}, {8.15392e-06, "Field Reading"=-2.384026805214854}, {8.63075e-06, "Field Reading"=-2.508800386025191}, {8.29697e-06, "Field Reading"=-2.3978503946337897}, {9.36985e-06, "Field Reading"=-2.6923773181538673}, {7.03335e-06, "Field Reading"=-2.0094539345681444}, {5.6982e-06, "Field Reading"=-1.61876083065822}, {6.58035e-06, "Field Reading"=-1.858813925109037}, {6.8903e-06, "Field Reading"=-1.9353524912716313}, {6.34193e-06, "Field Reading"=-1.7713849187617485}, {8.08239e-06, "Field Reading"=-2.244996083529157}, {5.93662e-06, "Field Reading"=-1.6398868552044947}, {6.91414e-06, "Field Reading"=-1.8994368286585532}, {6.00815e-06, "Field Reading"=-1.6415306727430201}, {5.76973e-06, "Field Reading"=-1.5677634278292392}, {6.03199e-06, "Field Reading"=-1.6301838554236405}, {8.44002e-06, "Field Reading"=-2.268718902630794}, {4.69685e-06, "Field Reading"=-1.2557952376114263}, {6.67572e-06, "Field Reading"=-1.775396063433977}, {5.29289e-06, "Field Reading"=-1.4002021115899357}, {5.10216e-06, "Field Reading"=-1.3425924220376135}, {6.29425e-06, "Field Reading"=-1.6476231610910421}, {5.67436e-06, "Field Reading"=-1.4776248050226681}, {5.45979e-06, "Field Reading"=-1.4143910760406924}, {4.41074e-06, "Field Reading"=-1.136741783843965}, {4.12464e-06, "Field Reading"=-1.0575647478417387}, {2.00272e-06, "Field Reading"=-0.5108849264049387}, {3.48091e-06, "Field Reading"=-0.8834281247541386}, {3.09944e-06, "Field Reading"=-0.7826473410433817}, {3.93391e-06, "Field Reading"=-0.9883724143822281}, {4.86374e-06, "Field Reading"=-1.2158802853871578}, {4.55379e-06, "Field Reading"=-1.1327441332888903}, {3.71933e-06, "Field Reading"=-0.9206034504096434}, {3.93391e-06, "Field Reading"=-0.9688860756999588}, {-2.14577e-07, "Field Reading"=0.05258969513824043}, {2.86102e-06, "Field Reading"=-0.6977825255599781}, {1.26362e-06, "Field Reading"=-0.30669420625077365}, {1.64509e-06, "Field Reading"=-0.39735513634936354}, {8.10623e-07, "Field Reading"=-0.19485801921602283}, {1.28746e-06, "Field Reading"=-0.30798710121906875}, {9.29832e-07, "Field Reading"=-0.22137697549175997}, {-4.76837e-08, "Field Reading"=0.011298946255974258}, {-1.19209e-07, "Field Reading"=0.028114335577750785}, {3.33786e-07, "Field Reading"=-0.07835131404749163}, {3.33786e-07, "Field Reading"=-0.07798556108502139}, {-7.39098e-07, "Field Reading"=0.17188045775998995}, {-1.07288e-06, "Field Reading"=0.24833977977922372}, {9.53674e-08, "Field Reading"=-0.021972992090244482}, {1.38283e-06, "Field Reading"=-0.31715047807768965}, {6.67572e-07, "Field Reading"=-0.15240882711511505}, {9.53674e-08, "Field Reading"=-0.021673867244227984}, {-2.09808e-06, "Field Reading"=0.4746712156142324}, {-1.50204e-06, "Field Reading"=0.3382805356491345}, {0.0, "Field Reading"=-0.0}, {-2.45571e-06, "Field Reading"=0.5481287540428152}, {-4.91142e-06, "Field Reading"=1.0913927122267308}, {-2.86102e-06, "Field Reading"=0.632946621358536}, {-2.45571e-06, "Field Reading"=0.5408921810264509}, {-3.14713e-06, "Field Reading"=0.6901222520695137}, {-4.3869e-06, "Field Reading"=0.9577903293066069}, {-3.3617e-06, "Field Reading"=0.7307741636758482}, {-4.48227e-06, "Field Reading"=0.9701505136163526}, {-1.14441e-06, "Field Reading"=0.24663158166959762}, {-3.88622e-06, "Field Reading"=0.8339313150734315}, {-3.43323e-06, "Field Reading"=0.7335820464991059}, {-5.17368e-06, "Field Reading"=1.1007267713989075}, {-4.14848e-06, "Field Reading"=0.8788780136434896}, {-4.81606e-06, "Field Reading"=1.0160078309262517}, {-5.03063e-06, "Field Reading"=1.0568195186716411}, {-5.79357e-06, "Field Reading"=1.2120084348993965}, {-3.24249e-06, "Field Reading"=0.6755018624534387}, {-5.81741e-06, "Field Reading"=1.2068664345906652}, {-5.38826e-06, "Field Reading"=1.113230858228999}, {-4.91142e-06, "Field Reading"=1.0105365817526402}, {-6.48499e-06, "Field Reading"=1.3288423787647177}, {-4.69685e-06, "Field Reading"=0.9585095180565533}, {-7.53403e-06, "Field Reading"=1.5312664502767201}, {-6.4373e-06, "Field Reading"=1.303020672875479}, {-6.98566e-06, "Field Reading"=1.4083310484976532}, {-7.10487e-06, "Field Reading"=1.4266205641930763}, {-9.05991e-06, "Field Reading"=1.8119131473004026}, {-7.89166e-06, "Field Reading"=1.5782751820934444}, {-6.8903e-06, "Field Reading"=1.3835332575669348}, {-7.7486e-06, "Field Reading"=1.5621421544118834}, {-5.79357e-06, "Field Reading"=1.1727233531770531}, {-5.98431e-06, "Field Reading"=1.2162910329605112}, {-5.26905e-06, "Field Reading"=1.07528340969154}, {-6.31809e-06, "Field Reading"=1.294642820551701}, {-5.74589e-06, "Field Reading"=1.182228376493245}, {-4.74453e-06, "Field Reading"=0.9802302374685447}, {-4.79221e-06, "Field Reading"=0.9941869993755487}, {-7.98702e-06, "Field Reading"=1.663927834836774}, {-5.53131e-06, "Field Reading"=1.1571463537602533}, {-6.03199e-06, "Field Reading"=1.267187519694799}, {-6.34193e-06, "Field Reading"=1.3379119314286194}, {-4.95911e-06, "Field Reading"=1.0506143807465786}, {-6.98566e-06, "Field Reading"=1.4862379075066539}, {-4.1008e-06, "Field Reading"=0.8762262102917264}, {-5.07832e-06, "Field Reading"=1.089742516807543}, {-5.76973e-06, "Field Reading"=1.243438775554186}, {-4.48227e-06, "Field Reading"=0.9701526134319732}, {-2.26498e-06, "Field Reading"=0.49236447901291464}, {-2.67029e-06, "Field Reading"=0.5830009278969488}, {-4.05312e-07, "Field Reading"=0.08887875305902271}, {-2.6226e-06, "Field Reading"=0.5776461130138872}, {-1.07288e-06, "Field Reading"=0.23735390483101299}, {-2.98023e-06, "Field Reading"=0.662246843459595}, {-1.33514e-06, "Field Reading"=0.2980076871225074}, {-2.7895e-06, "Field Reading"=0.6254133736898156}, {-2.24113e-06, "Field Reading"=0.5047283160708695}, {-2.19345e-06, "Field Reading"=0.4962410607832802}, {-1.85966e-06, "Field Reading"=0.4226355919684556}, {-3.88622e-06, "Field Reading"=0.8872243276562713}, {-3.98159e-06, "Field Reading"=0.9131626385824569}, {-1.85966e-06, "Field Reading"=0.42846939339760015}, {-2.16961e-06, "Field Reading"=0.502195474798912}, {-2.59876e-06, "Field Reading"=0.604347330649681}, {1.00136e-06, "Field Reading"=-0.233955510697105}, {-1.43051e-07, "Field Reading"=0.03357878577330429}, {-6.19888e-07, "Field Reading"=0.14619379365970311}, {-2.86102e-07, "Field Reading"=0.06779314822450014}, {-7.15256e-08, "Field Reading"=0.017028891137432296}, {-1.90735e-07, "Field Reading"=0.04562743554842151}, {2.02656e-06, "Field Reading"=-0.487142136006346}, {3.33786e-06, "Field Reading"=-0.8062210606913309}, {2.67029e-06, "Field Reading"=-0.6481050447192457}, {1.90735e-06, "Field Reading"=-0.46518689423391174}, {2.81334e-06, "Field Reading"=-0.6895069383513635}, {5.26905e-06, "Field Reading"=-1.2977156579028386}, {2.24113e-06, "Field Reading"=-0.5547186717226221}, {3.24249e-06, "Field Reading"=-0.8065614630336256}, {1.81198e-06, "Field Reading"=-0.45297574853068745}, {3.48091e-06, "Field Reading"=-0.8745631468002623}, {5.55515e-06, "Field Reading"=-1.4027412687711005}, {4.22001e-06, "Field Reading"=-1.0710032891397478}, {3.95775e-06, "Field Reading"=-1.0096017713788645}, {4.74453e-06, "Field Reading"=-1.216505603659365}, {5.74589e-06, "Field Reading"=-1.4808384190342665}, {4.3869e-06, "Field Reading"=-1.1364495956147123}, {3.86238e-06, "Field Reading"=-1.0057757408468309}, {4.19617e-06, "Field Reading"=-1.098416313282027}, {3.21865e-06, "Field Reading"=-0.846961894411654}, {7.51019e-06, "Field Reading"=-1.9867754471454382}, {3.50475e-06, "Field Reading"=-0.9320821354580826}, {5.88894e-06, "Field Reading"=-1.574528158112151}, {3.86238e-06, "Field Reading"=-1.0382267477023899}, {5.17368e-06, "Field Reading"=-1.398220091400712}, {4.79221e-06, "Field Reading"=-1.3021495939112502}, {6.05583e-06, "Field Reading"=-1.6545576748112751}, {6.12736e-06, "Field Reading"=-1.6832990393094676}, {6.7234e-06, "Field Reading"=-1.857220991453369}, {7.55787e-06, "Field Reading"=-2.099303368164925}, {8.4877e-06, "Field Reading"=-2.3707202350693533}, {7.96318e-06, "Field Reading"=-2.236710090949436}, {8.74996e-06, "Field Reading"=-2.4716842557230345}, {8.86917e-06, "Field Reading"=-2.519586146945106}, {9.15527e-06, "Field Reading"=-2.6156868010993843}, {7.29561e-06, "Field Reading"=-2.096355319038889}, {8.13007e-06, "Field Reading"=-2.3496157703234233}, {9.34601e-06, "Field Reading"=-2.7166975271858407}, {1.02043e-05, "Field Reading"=-2.983512804694421}, {8.98838e-06, "Field Reading"=-2.643578974612362}, {9.60827e-06, "Field Reading"=-2.8425993313807285}, {9.70364e-06, "Field Reading"=-2.8878849564896494}, {1.12057e-05, "Field Reading"=-3.354849333113782}, {1.02043e-05, "Field Reading"=-3.073417706268937}, {1.08719e-05, "Field Reading"=-3.294335460490034}, {8.51154e-06, "Field Reading"=-2.594950061584615}, {1.09196e-05, "Field Reading"=-3.3494986303975067}, {1.11341e-05, "Field Reading"=-3.436344557266751}, {1.24693e-05, "Field Reading"=-3.8722730307594366}, {1.21355e-05, "Field Reading"=-3.792154142292885}, {1.2064e-05, "Field Reading"=-3.793484037117279}, {1.32561e-05, "Field Reading"=-4.194915254237288}, {1.21117e-05, "Field Reading"=-3.8571801633100216}, {1.41859e-05, "Field Reading"=-4.546660812097165}, {1.42574e-05, "Field Reading"=-4.599027770161512}, {1.31607e-05, "Field Reading"=-4.272801945385067}, {1.42097e-05, "Field Reading"=-4.643495537771271}, {1.49488e-05, "Field Reading"=-4.917109625809168}, {1.39713e-05, "Field Reading"=-4.626197004013192}, {1.41859e-05, "Field Reading"=-4.728523001129974}, {1.34945e-05, "Field Reading"=-4.528203751551961}, {1.33514e-05, "Field Reading"=-4.510425253030283}, {1.23024e-05, "Field Reading"=-4.1843047756391725}, {1.33753e-05, "Field Reading"=-4.580346899988014}, {1.56879e-05, "Field Reading"=-5.4095833821835715}, {1.28746e-05, "Field Reading"=-4.470285134928681}, {1.66178e-05, "Field Reading"=-5.810277370833581}, {1.31369e-05, "Field Reading"=-4.6255061441498535}, {1.53542e-05, "Field Reading"=-5.44452009134363}, {1.56641e-05, "Field Reading"=-5.59408168221362}, {1.72138e-05, "Field Reading"=-6.192036662002383}, {1.8096e-05, "Field Reading"=-6.5564742284476205}, {1.89543e-05, "Field Reading"=-6.91750150544698}, {1.688e-05, "Field Reading"=-6.2056998323578725}, {1.719e-05, "Field Reading"=-6.366430872930632}, {1.61409e-05, "Field Reading"=-6.02238680670858}, {1.88589e-05, "Field Reading"=-7.0893323008217495}, {1.76191e-05, "Field Reading"=-6.673800396963682}, {1.85728e-05, "Field Reading"=-7.088746736691042}, {1.73092e-05, "Field Reading"=-6.657205382931998}, {1.92404e-05, "Field Reading"=-7.457230339909305}, {1.94788e-05, "Field Reading"=-7.608549599237536}, {1.81675e-05, "Field Reading"=-7.152136684841445}, {1.77622e-05, "Field Reading"=-7.048464093396455}, {1.63078e-05, "Field Reading"=-6.523067815457477}, {1.85251e-05, "Field Reading"=-7.469617670540229}, {2.05755e-05, "Field Reading"=-8.36385439320339}, {1.90973e-05, "Field Reading"=-7.82653776326089}, {1.96695e-05, "Field Reading"=-8.127489545972926}, {1.95503e-05, "Field Reading"=-8.145992274967814}, {1.82152e-05, "Field Reading"=-7.653381064024672}, {1.94073e-05, "Field Reading"=-8.223292825545329}, {2.04802e-05, "Field Reading"=-8.7520352129228}, {2.02656e-05, "Field Reading"=-8.734871211337541}, {2.04086e-05, "Field Reading"=-8.872879992696001}, {2.05278e-05, "Field Reading"=-9.002947213304562}, {2.17438e-05, "Field Reading"=-9.621150442477877}, {2.10285e-05, "Field Reading"=-9.387597487533649}, {2.12193e-05, "Field Reading"=-9.558071025747282}, {2.26974e-05, "Field Reading"=-10.31671863494632}, {2.19584e-05, "Field Reading"=-10.072244723841678}, {2.29597e-05, "Field Reading"=-10.628998657469563}, {2.43902e-05, "Field Reading"=-11.397396237348012}, {2.41756e-05, "Field Reading"=-11.403746279428482}, {2.35796e-05, "Field Reading"=-11.228380952380954}, {2.57254e-05, "Field Reading"=-12.367742928020617}, {2.34127e-05, "Field Reading"=-11.364891825114436}, {2.36988e-05, "Field Reading"=-11.61643244727}, {2.18391e-05, "Field Reading"=-10.81164973563833}, {2.4724e-05, "Field Reading"=-12.36206181030905}, {2.50578e-05, "Field Reading"=-12.655326713871577}, {2.49624e-05, "Field Reading"=-12.735463529363747}, {2.43902e-05, "Field Reading"=-12.57174961857243}, {3.61204e-05, "Field Reading"=-18.811630583664478}, {3.75986e-05, "Field Reading"=-19.787487106077513}, {3.59297e-05, "Field Reading"=-19.111745869636913}, {3.57628e-05, "Field Reading"=-19.227311827956992}, {3.53575e-05, "Field Reading"=-19.2159281743034}, {3.4523e-05, "Field Reading"=-18.967951782074316}, {3.44992e-05, "Field Reading"=-19.16537042798098}, {3.36885e-05, "Field Reading"=-18.925060389865738}, {3.43084e-05, "Field Reading"=-19.49418442778974}, {3.75509e-05, "Field Reading"=-21.581473137313502}, {3.59058e-05, "Field Reading"=-20.875829229579583}, {3.36647e-05, "Field Reading"=-19.80253173492077}, {3.42846e-05, "Field Reading"=-20.40713558686452}, {3.30687e-05, "Field Reading"=-19.92030360531309}, {3.407e-05, "Field Reading"=-20.77553036447122}, {3.37601e-05, "Field Reading"=-20.84021111762709}, {3.55005e-05, "Field Reading"=-22.18878325926759}, {3.25203e-05, "Field Reading"=-20.582989442770703}, {3.39031e-05, "Field Reading"=-21.7331743559171}, {3.35217e-05, "Field Reading"=-21.76747900960396}, {3.35932e-05, "Field Reading"=-22.100644074710036}, {3.2711e-05, "Field Reading"=-21.80922346603372}, {3.6025e-05, "Field Reading"=-24.3428610041219}, {3.37601e-05, "Field Reading"=-23.124464871603436}, {3.32594e-05, "Field Reading"=-23.098249196130315}, {3.53336e-05, "Field Reading"=-24.88369308778478}, {3.4523e-05, "Field Reading"=-24.659814138874406}, {3.52859e-05, "Field Reading"=-25.572643006747207}, {3.50952e-05, "Field Reading"=-25.807761035981382}, {3.55721e-05, "Field Reading"=-26.548324501828493}, {3.5429e-05, "Field Reading"=-26.841371577495945}, {3.37362e-05, "Field Reading"=-25.95152195819903}, {3.41654e-05, "Field Reading"=-26.691927280681885}, {3.30448e-05, "Field Reading"=-26.229570656358398}, {3.30925e-05, "Field Reading"=-26.690943992773263}, {3.16143e-05, "Field Reading"=-25.916122209743662}, {3.28064e-05, "Field Reading"=-27.3407172204582}, {3.29971e-05, "Field Reading"=-27.965303026450727}, {3.32117e-05, "Field Reading"=-28.63176316424704}, {3.21388e-05, "Field Reading"=-28.192177124360736}, {3.49283e-05, "Field Reading"=-31.19071644803229}, {3.39985e-05, "Field Reading"=-30.912223596159443}, {3.04937e-05, "Field Reading"=-28.238306462814965}, {3.1805e-05, "Field Reading"=-30.007547881875645}, {3.36885e-05, "Field Reading"=-32.39465738407985}, {3.3617e-05, "Field Reading"=-32.95881251409355}, {3.42846e-05, "Field Reading"=-34.28573142913716}, {3.46899e-05, "Field Reading"=-35.398507319522196}, {3.51191e-05, "Field Reading"=-36.58365339641883}, {3.44992e-05, "Field Reading"=-36.7023308116297}, {3.46661e-05, "Field Reading"=-37.68123976203908}, {3.6335e-05, "Field Reading"=-40.37347828599111}, {3.36885e-05, "Field Reading"=-38.28303891543606}, {3.46184e-05, "Field Reading"=-40.25526412487849}, {3.49045e-05, "Field Reading"=-41.55391610048322}, {3.55482e-05, "Field Reading"=-43.3519920974646}, {3.29018e-05, "Field Reading"=-41.128278206955166}, {3.45945e-05, "Field Reading"=-44.352605424698844}, {3.45469e-05, "Field Reading"=-45.456866050082034}, {3.56436e-05, "Field Reading"=-48.16754775727305}, {3.27587e-05, "Field Reading"=-45.498510406322275}, {3.49998e-05, "Field Reading"=-50.00064286908186}, {3.54052e-05, "Field Reading"=-52.06685343274582}, {3.6335e-05, "Field Reading"=-55.0530303030303}, {3.407e-05, "Field Reading"=-53.23578907564732}, {3.37362e-05, "Field Reading"=-54.413752391152165}, {3.36885e-05, "Field Reading"=-56.1474064209893}, {3.26395e-05, "Field Reading"=-56.27606730472475}, {3.54767e-05, "Field Reading"=-63.352381292523084}, {3.23057e-05, "Field Reading"=-59.82548115829844}, {3.2258e-05, "Field Reading"=-62.03628559230441}, {3.26872e-05, "Field Reading"=-65.37466149864599}, {3.21627e-05, "Field Reading"=-67.0078585952865}, {3.10183e-05, "Field Reading"=-67.43328586801744}, {3.33548e-05, "Field Reading"=-75.80825884283472}, {3.14236e-05, "Field Reading"=-74.82183632991173}, {3.19481e-05, "Field Reading"=-79.87444340827894}, {3.21627e-05, "Field Reading"=-84.64247084738001}, {3.04222e-05, "Field Reading"=-84.51315387393394}, {3.19958e-05, "Field Reading"=-94.11276777861772}, {3.24965e-05, "Field Reading"=-101.56425803225403}, {3.28541e-05, "Field Reading"=-109.52717501825225}, {3.1805e-05, "Field Reading"=-113.60226883072352}, {3.03268e-05, "Field Reading"=-116.66083236843016}, {2.97546e-05, "Field Reading"=-123.99868310836435}, {3.1662e-05, "Field Reading"=-143.94304470772227}, {3.09467e-05, "Field Reading"=-154.77296710661219}, {3.01123e-05, "Field Reading"=-167.33703806612948}, {3.03984e-05, "Field Reading"=-190.06959164149987}, {3.24249e-05, "Field Reading"=-231.70904257599796}, {3.14474e-05, "Field Reading"=-262.18620511409586}, {2.95639e-05, "Field Reading"=-295.6455042010924}, {3.02553e-05, "Field Reading"=-378.18841358689815}, {3.19958e-05, "Field Reading"=-533.2588895092542}, {3.08275e-05, "Field Reading"=-770.7086944890985}, {3.16381e-05, "Field Reading"=-1582.1660573994707}, {2.89917e-05, "Field Reading"=6608698.625453053}]
  in  "Wait (ms)":u32=50
  out "Voltage (V)":dbl=2.89917e-05 format="%#_13g"
  in  "Set Compliance voltage (V)":dbl=1.0 min=0.0 step=0.1 format="%_3f"
  out "Current (A)":dbl=4.3869e-12
  in  "Folder":path=path "D:/Pranava/Data/PtTe2/29-10-2022/002"
  out "I vs V":cluster{dbl, "Field Reading":dbl}[](graph)=[{3.33548e-05, "Field Reading"=4.41074e-13}, {3.15428e-05, "Field Reading"=2.00023e-08}, {3.19242e-05, "Field Reading"=4.00057e-08}, {3.13759e-05, "Field Reading"=6.00064e-08}, {3.35217e-05, "Field Reading"=8.00077e-08}, {3.21865e-05, "Field Reading"=1.00008e-07}, {3.17812e-05, "Field Reading"=1.20037e-07}, {3.32117e-05, "Field Reading"=1.40028e-07}, {3.36409e-05, "Field Reading"=1.60038e-07}, {3.27587e-05, "Field Reading"=1.80054e-07}, {3.33786e-05, "Field Reading"=2.00048e-07}, {3.28064e-05, "Field Reading"=2.20056e-07}, {3.19719e-05, "Field Reading"=2.40046e-07}, {3.27826e-05, "Field Reading"=2.60055e-07}, {3.20911e-05, "Field Reading"=2.80048e-07}, {3.31402e-05, "Field Reading"=3.00061e-07}, {3.37124e-05, "Field Reading"=3.20052e-07}, {3.19719e-05, "Field Reading"=3.40068e-07}, {3.04937e-05, "Field Reading"=3.60086e-07}, {3.25918e-05, "Field Reading"=3.80076e-07}, {3.10421e-05, "Field Reading"=4.00083e-07}, {3.25918e-05, "Field Reading"=4.20077e-07}, {3.25441e-05, "Field Reading"=4.40084e-07}, {3.20196e-05, "Field Reading"=4.60073e-07}, {3.03268e-05, "Field Reading"=4.80084e-07}, {3.09229e-05, "Field Reading"=5.00104e-07}, {2.90155e-05, "Field Reading"=5.2009e-07}, {3.00884e-05, "Field Reading"=5.40096e-07}, {2.91348e-05, "Field Reading"=5.60091e-07}, {3.13044e-05, "Field Reading"=5.80102e-07}, {3.03507e-05, "Field Reading"=6.00093e-07}, {3.16858e-05, "Field Reading"=6.20105e-07}, {2.99692e-05, "Field Reading"=6.40095e-07}, {3.11136e-05, "Field Reading"=6.60111e-07}, {2.86102e-05, "Field Reading"=6.80119e-07}, {2.87533e-05, "Field Reading"=7.00107e-07}, {2.96354e-05, "Field Reading"=7.20114e-07}, {2.9397e-05, "Field Reading"=7.40111e-07}, {2.84672e-05, "Field Reading"=7.60116e-07}, {3.11852e-05, "Field Reading"=7.80104e-07}, {3.11375e-05, "Field Reading"=8.00116e-07}, {3.05891e-05, "Field Reading"=8.20101e-07}, {2.89917e-05, "Field Reading"=8.40112e-07}, {2.94447e-05, "Field Reading"=8.60121e-07}, {2.97546e-05, "Field Reading"=8.80109e-07}, {3.3474e-05, "Field Reading"=9.00116e-07}, {3.24249e-05, "Field Reading"=9.20108e-07}, {3.03745e-05, "Field Reading"=9.40113e-07}, {3.14236e-05, "Field Reading"=9.60105e-07}, {3.10183e-05, "Field Reading"=9.80107e-07}, {3.16858e-05, "Field Reading"=1.00011e-06}, {3.33786e-05, "Field Reading"=1.02013e-06}, {3.29733e-05, "Field Reading"=1.04009e-06}, {3.20911e-05, "Field Reading"=1.06006e-06}, {3.47137e-05, "Field Reading"=1.08004e-06}, {3.34263e-05, "Field Reading"=1.10017e-06}, {3.31163e-05, "Field Reading"=1.12016e-06}, {3.33548e-05, "Field Reading"=1.14013e-06}, {3.34263e-05, "Field Reading"=1.16011e-06}, {2.95877e-05, "Field Reading"=1.18007e-06}, {3.04461e-05, "Field Reading"=1.20004e-06}, {3.06368e-05, "Field Reading"=1.22019e-06}, {3.06606e-05, "Field Reading"=1.24015e-06}, {3.10898e-05, "Field Reading"=1.26011e-06}, {3.18766e-05, "Field Reading"=1.28012e-06}, {3.20196e-05, "Field Reading"=1.30009e-06}, {3.20911e-05, "Field Reading"=1.32023e-06}, {3.09706e-05, "Field Reading"=1.3402e-06}, {3.23057e-05, "Field Reading"=1.36016e-06}, {3.05414e-05, "Field Reading"=1.38014e-06}, {3.20196e-05, "Field Reading"=1.4001e-06}, {3.19719e-05, "Field Reading"=1.42006e-06}, {3.25918e-05, "Field Reading"=1.4402e-06}, {3.37362e-05, "Field Reading"=1.46019e-06}, {3.12805e-05, "Field Reading"=1.48016e-06}, {3.00407e-05, "Field Reading"=1.50012e-06}, {2.97308e-05, "Field Reading"=1.5201e-06}, {3.01838e-05, "Field Reading"=1.54024e-06}, {3.09944e-05, "Field Reading"=1.5602e-06}, {3.03745e-05, "Field Reading"=1.58017e-06}, {3.02315e-05, "Field Reading"=1.60015e-06}, {3.01838e-05, "Field Reading"=1.62013e-06}, {3.02315e-05, "Field Reading"=1.64009e-06}, {3.21388e-05, "Field Reading"=1.66021e-06}, {3.12805e-05, "Field Reading"=1.68019e-06}, {2.99454e-05, "Field Reading"=1.70017e-06}, {3.31879e-05, "Field Reading"=1.72015e-06}, {3.3021e-05, "Field Reading"=1.74013e-06}, {3.1352e-05, "Field Reading"=1.76027e-06}, {3.12805e-05, "Field Reading"=1.78023e-06}, {3.20435e-05, "Field Reading"=1.80023e-06}, {3.23057e-05, "Field Reading"=1.82019e-06}, {3.35693e-05, "Field Reading"=1.84017e-06}, {3.11613e-05, "Field Reading"=1.86015e-06}, {3.07322e-05, "Field Reading"=1.88029e-06}, {3.22819e-05, "Field Reading"=1.90026e-06}, {3.32356e-05, "Field Reading"=1.92023e-06}, {3.12805e-05, "Field Reading"=1.9402e-06}, {3.08514e-05, "Field Reading"=1.9602e-06}, {3.02553e-05, "Field Reading"=1.98034e-06}, {2.97546e-05, "Field Reading"=2.00031e-06}, {3.06845e-05, "Field Reading"=2.02026e-06}, {3.32356e-05, "Field Reading"=2.04023e-06}, {3.25203e-05, "Field Reading"=2.0602e-06}, {3.14951e-05, "Field Reading"=2.08017e-06}, {3.14236e-05, "Field Reading"=2.10028e-06}, {3.09467e-05, "Field Reading"=2.12024e-06}, {3.08752e-05, "Field Reading"=2.14025e-06}, {2.91109e-05, "Field Reading"=2.16022e-06}, {3.0756e-05, "Field Reading"=2.1802e-06}, {3.11613e-05, "Field Reading"=2.20034e-06}, {3.13282e-05, "Field Reading"=2.22032e-06}, {3.24011e-05, "Field Reading"=2.24031e-06}, {3.09706e-05, "Field Reading"=2.26026e-06}, {3.32594e-05, "Field Reading"=2.28023e-06}, {3.12567e-05, "Field Reading"=2.30022e-06}, {3.10898e-05, "Field Reading"=2.32036e-06}, {3.07798e-05, "Field Reading"=2.34034e-06}, {3.32117e-05, "Field Reading"=2.3603e-06}, {3.18289e-05, "Field Reading"=2.38027e-06}, {3.18289e-05, "Field Reading"=2.40026e-06}, {3.46661e-05, "Field Reading"=2.42039e-06}, {3.24726e-05, "Field Reading"=2.44034e-06}, {3.2711e-05, "Field Reading"=2.46031e-06}, {3.23772e-05, "Field Reading"=2.48029e-06}, {3.49998e-05, "Field Reading"=2.50027e-06}, {3.3164e-05, "Field Reading"=2.52024e-06}, {3.22104e-05, "Field Reading"=2.54036e-06}, {3.3164e-05, "Field Reading"=2.56033e-06}, {3.53336e-05, "Field Reading"=2.58031e-06}, {3.56197e-05, "Field Reading"=2.60027e-06}, {3.41654e-05, "Field Reading"=2.62023e-06}, {3.438e-05, "Field Reading"=2.6404e-06}, {3.28064e-05, "Field Reading"=2.66036e-06}, {3.47137e-05, "Field Reading"=2.68034e-06}, {3.28302e-05, "Field Reading"=2.70029e-06}, {5.20706e-05, "Field Reading"=2.72026e-06}, {5.3215e-05, "Field Reading"=2.74022e-06}, {5.37634e-05, "Field Reading"=2.76036e-06}, {5.20945e-05, "Field Reading"=2.78033e-06}, {5.32627e-05, "Field Reading"=2.80031e-06}, {5.1713e-05, "Field Reading"=2.8203e-06}, {5.22375e-05, "Field Reading"=2.84028e-06}, {5.36203e-05, "Field Reading"=2.8604e-06}, {5.35727e-05, "Field Reading"=2.88037e-06}, {5.24282e-05, "Field Reading"=2.90035e-06}, {5.28336e-05, "Field Reading"=2.92033e-06}, {5.27859e-05, "Field Reading"=2.94029e-06}, {5.31435e-05, "Field Reading"=2.96026e-06}, {5.19037e-05, "Field Reading"=2.98042e-06}, {5.29528e-05, "Field Reading"=3.00038e-06}, {5.46932e-05, "Field Reading"=3.02036e-06}, {5.49078e-05, "Field Reading"=3.04033e-06}, {5.23329e-05, "Field Reading"=3.06029e-06}, {5.56707e-05, "Field Reading"=3.08045e-06}, {5.28812e-05, "Field Reading"=3.10042e-06}, {5.53131e-05, "Field Reading"=3.12039e-06}, {5.43594e-05, "Field Reading"=3.14037e-06}, {5.45979e-05, "Field Reading"=3.16035e-06}, {5.47171e-05, "Field Reading"=3.18032e-06}, {5.50985e-05, "Field Reading"=3.20046e-06}, {5.63622e-05, "Field Reading"=3.22044e-06}, {5.61714e-05, "Field Reading"=3.24041e-06}, {5.70059e-05, "Field Reading"=3.26038e-06}, {5.66244e-05, "Field Reading"=3.28035e-06}, {5.7292e-05, "Field Reading"=3.30048e-06}, {5.6839e-05, "Field Reading"=3.32046e-06}, {5.6076e-05, "Field Reading"=3.34044e-06}, {5.76735e-05, "Field Reading"=3.3604e-06}, {5.94378e-05, "Field Reading"=3.38037e-06}, {5.65767e-05, "Field Reading"=3.40035e-06}, {5.73397e-05, "Field Reading"=3.42048e-06}, {5.84126e-05, "Field Reading"=3.44045e-06}, {5.8651e-05, "Field Reading"=3.46042e-06}, {5.5933e-05, "Field Reading"=3.48037e-06}, {5.68867e-05, "Field Reading"=3.50038e-06}, {5.94139e-05, "Field Reading"=3.52051e-06}, {5.85318e-05, "Field Reading"=3.54049e-06}, {5.99623e-05, "Field Reading"=3.56045e-06}, {6.00338e-05, "Field Reading"=3.58043e-06}, {6.00576e-05, "Field Reading"=3.6004e-06}, {6.03437e-05, "Field Reading"=3.62037e-06}, {6.06775e-05, "Field Reading"=3.6405e-06}, {5.86271e-05, "Field Reading"=3.66047e-06}, {6.02484e-05, "Field Reading"=3.68047e-06}, {6.00576e-05, "Field Reading"=3.70044e-06}, {6.08444e-05, "Field Reading"=3.72042e-06}, {6.02961e-05, "Field Reading"=3.74055e-06}, {6.001e-05, "Field Reading"=3.76052e-06}, {6.31094e-05, "Field Reading"=3.78049e-06}, {6.26802e-05, "Field Reading"=3.80047e-06}, {6.08444e-05, "Field Reading"=3.82046e-06}, {6.19412e-05, "Field Reading"=3.84044e-06}, {6.21319e-05, "Field Reading"=3.86058e-06}, {6.39439e-05, "Field Reading"=3.88054e-06}, {6.33001e-05, "Field Reading"=3.90052e-06}, {6.20842e-05, "Field Reading"=3.92048e-06}, {6.41823e-05, "Field Reading"=3.94044e-06}, {6.37531e-05, "Field Reading"=3.96058e-06}, {6.51598e-05, "Field Reading"=3.98055e-06}, {6.55174e-05, "Field Reading"=4.00053e-06}, {6.50883e-05, "Field Reading"=4.02053e-06}, {6.44922e-05, "Field Reading"=4.04049e-06}, {6.49452e-05, "Field Reading"=4.06045e-06}, {6.64234e-05, "Field Reading"=4.08058e-06}, {6.43253e-05, "Field Reading"=4.10053e-06}, {6.5732e-05, "Field Reading"=4.12049e-06}, {6.71148e-05, "Field Reading"=4.14046e-06}, {6.58512e-05, "Field Reading"=4.16044e-06}, {6.46591e-05, "Field Reading"=4.1806e-06}, {6.61135e-05, "Field Reading"=4.20057e-06}, {6.44922e-05, "Field Reading"=4.22054e-06}, {6.61612e-05, "Field Reading"=4.2405e-06}, {6.61135e-05, "Field Reading"=4.26047e-06}, {6.53028e-05, "Field Reading"=4.28044e-06}, {6.53744e-05, "Field Reading"=4.30058e-06}, {6.59227e-05, "Field Reading"=4.32053e-06}, {6.62088e-05, "Field Reading"=4.3405e-06}, {6.58035e-05, "Field Reading"=4.36049e-06}, {6.51598e-05, "Field Reading"=4.38045e-06}, {6.6185e-05, "Field Reading"=4.40059e-06}, {6.44922e-05, "Field Reading"=4.42055e-06}, {6.62088e-05, "Field Reading"=4.44053e-06}, {6.67334e-05, "Field Reading"=4.46052e-06}, {6.73532e-05, "Field Reading"=4.4805e-06}, {6.75201e-05, "Field Reading"=4.50046e-06}, {6.7687e-05, "Field Reading"=4.52061e-06}, {6.74486e-05, "Field Reading"=4.54059e-06}, {6.63996e-05, "Field Reading"=4.56055e-06}, {6.4683e-05, "Field Reading"=4.58053e-06}, {6.57082e-05, "Field Reading"=4.60051e-06}, {6.5732e-05, "Field Reading"=4.62064e-06}, {6.73771e-05, "Field Reading"=4.64059e-06}, {6.92368e-05, "Field Reading"=4.66055e-06}, {6.73771e-05, "Field Reading"=4.68051e-06}, {6.82592e-05, "Field Reading"=4.7005e-06}, {6.88076e-05, "Field Reading"=4.72063e-06}, {6.62565e-05, "Field Reading"=4.74059e-06}, {6.82831e-05, "Field Reading"=4.76056e-06}, {6.65903e-05, "Field Reading"=4.78052e-06}, {6.88076e-05, "Field Reading"=4.8005e-06}, {6.85453e-05, "Field Reading"=4.82046e-06}, {6.48737e-05, "Field Reading"=4.8406e-06}, {6.90699e-05, "Field Reading"=4.86059e-06}, {7.12872e-05, "Field Reading"=4.88056e-06}, {6.96421e-05, "Field Reading"=4.90053e-06}, {7.20501e-05, "Field Reading"=4.9205e-06}, {7.27654e-05, "Field Reading"=4.94063e-06}, {7.08103e-05, "Field Reading"=4.9606e-06}, {7.32422e-05, "Field Reading"=4.98057e-06}, {7.10487e-05, "Field Reading"=5.00053e-06}, {7.09057e-05, "Field Reading"=5.00054e-06}, {7.0262e-05, "Field Reading"=4.98057e-06}, {7.00235e-05, "Field Reading"=4.96059e-06}, {7.04288e-05, "Field Reading"=4.94064e-06}, {7.01189e-05, "Field Reading"=4.92051e-06}, {7.08103e-05, "Field Reading"=4.90054e-06}, {6.99759e-05, "Field Reading"=4.88055e-06}, {7.02143e-05, "Field Reading"=4.86059e-06}, {7.15733e-05, "Field Reading"=4.84059e-06}, {7.06196e-05, "Field Reading"=4.82045e-06}, {7.11679e-05, "Field Reading"=4.8005e-06}, {6.81162e-05, "Field Reading"=4.78052e-06}, {6.71864e-05, "Field Reading"=4.76055e-06}, {6.73532e-05, "Field Reading"=4.74058e-06}, {6.7234e-05, "Field Reading"=4.72059e-06}, {6.69956e-05, "Field Reading"=4.70047e-06}, {6.69718e-05, "Field Reading"=4.68049e-06}, {6.87599e-05, "Field Reading"=4.66052e-06}, {6.73294e-05, "Field Reading"=4.64056e-06}, {6.65903e-05, "Field Reading"=4.62059e-06}, {6.28948e-05, "Field Reading"=4.60045e-06}, {6.51121e-05, "Field Reading"=4.58048e-06}, {6.77824e-05, "Field Reading"=4.56051e-06}, {6.72102e-05, "Field Reading"=4.54055e-06}, {6.58989e-05, "Field Reading"=4.52058e-06}, {6.60658e-05, "Field Reading"=4.50044e-06}, {6.79493e-05, "Field Reading"=4.48048e-06}, {6.61612e-05, "Field Reading"=4.4605e-06}, {6.77347e-05, "Field Reading"=4.44052e-06}, {6.49214e-05, "Field Reading"=4.42053e-06}, {6.53744e-05, "Field Reading"=4.40057e-06}, {6.54936e-05, "Field Reading"=4.38044e-06}, {6.3777e-05, "Field Reading"=4.36046e-06}, {6.48737e-05, "Field Reading"=4.34047e-06}, {6.44922e-05, "Field Reading"=4.32049e-06}, {6.34193e-05, "Field Reading"=4.30053e-06}, {6.45399e-05, "Field Reading"=4.2804e-06}, {6.3014e-05, "Field Reading"=4.26042e-06}, {6.42538e-05, "Field Reading"=4.24044e-06}, {6.6185e-05, "Field Reading"=4.22048e-06}, {6.60658e-05, "Field Reading"=4.20052e-06}, {6.51598e-05, "Field Reading"=4.18054e-06}, {6.46353e-05, "Field Reading"=4.16041e-06}, {6.57082e-05, "Field Reading"=4.14043e-06}, {6.36101e-05, "Field Reading"=4.12046e-06}, {6.30617e-05, "Field Reading"=4.10049e-06}, {6.22272e-05, "Field Reading"=4.08052e-06}, {6.17981e-05, "Field Reading"=4.06039e-06}, {6.36339e-05, "Field Reading"=4.04043e-06}, {6.23465e-05, "Field Reading"=4.02047e-06}, {6.19888e-05, "Field Reading"=4.00048e-06}, {6.07967e-05, "Field Reading"=3.9805e-06}, {6.16312e-05, "Field Reading"=3.96054e-06}, {6.22749e-05, "Field Reading"=3.9404e-06}, {6.32763e-05, "Field Reading"=3.92044e-06}, {6.21557e-05, "Field Reading"=3.90049e-06}, {6.32048e-05, "Field Reading"=3.88052e-06}, {6.53744e-05, "Field Reading"=3.86055e-06}, {6.43969e-05, "Field Reading"=3.84041e-06}, {6.08206e-05, "Field Reading"=3.82042e-06}, {6.02484e-05, "Field Reading"=3.80044e-06}, {6.33001e-05, "Field Reading"=3.78048e-06}, {6.1655e-05, "Field Reading"=3.7605e-06}, {6.02484e-05, "Field Reading"=3.74052e-06}, {6.1655e-05, "Field Reading"=3.72039e-06}, {6.13689e-05, "Field Reading"=3.70042e-06}, {5.96762e-05, "Field Reading"=3.68044e-06}, {6.10828e-05, "Field Reading"=3.66046e-06}, {6.04391e-05, "Field Reading"=3.64049e-06}, {6.29902e-05, "Field Reading"=3.62035e-06}, {6.03914e-05, "Field Reading"=3.60039e-06}, {5.93424e-05, "Field Reading"=3.58042e-06}, {6.05345e-05, "Field Reading"=3.56045e-06}, {5.87702e-05, "Field Reading"=3.54049e-06}, {5.83649e-05, "Field Reading"=3.52052e-06}, {6.07014e-05, "Field Reading"=3.50038e-06}, {5.79834e-05, "Field Reading"=3.48036e-06}, {6.0606e-05, "Field Reading"=3.46041e-06}, {5.97239e-05, "Field Reading"=3.44045e-06}, {5.9557e-05, "Field Reading"=3.42047e-06}, {5.98431e-05, "Field Reading"=3.40034e-06}, {5.81503e-05, "Field Reading"=3.38035e-06}, {5.89848e-05, "Field Reading"=3.3604e-06}, {5.88655e-05, "Field Reading"=3.34042e-06}, {5.87702e-05, "Field Reading"=3.32046e-06}, {5.79834e-05, "Field Reading"=3.30047e-06}, {5.3525e-05, "Field Reading"=3.28034e-06}, {5.47409e-05, "Field Reading"=3.26037e-06}, {5.61237e-05, "Field Reading"=3.24041e-06}, {5.73635e-05, "Field Reading"=3.22043e-06}, {5.7888e-05, "Field Reading"=3.20046e-06}, {5.66244e-05, "Field Reading"=3.18032e-06}, {5.72443e-05, "Field Reading"=3.16035e-06}, {5.68151e-05, "Field Reading"=3.14036e-06}, {5.86271e-05, "Field Reading"=3.12039e-06}, {5.83887e-05, "Field Reading"=3.10041e-06}, {5.54085e-05, "Field Reading"=3.08044e-06}, {5.68628e-05, "Field Reading"=3.0603e-06}, {5.68151e-05, "Field Reading"=3.04034e-06}, {5.65052e-05, "Field Reading"=3.02035e-06}, {5.56231e-05, "Field Reading"=3.00039e-06}, {5.50032e-05, "Field Reading"=2.98043e-06}, {5.42879e-05, "Field Reading"=2.96026e-06}, {5.49793e-05, "Field Reading"=2.94029e-06}, {5.19753e-05, "Field Reading"=2.92031e-06}, {5.30243e-05, "Field Reading"=2.90034e-06}, {5.31197e-05, "Field Reading"=2.88035e-06}, {5.33104e-05, "Field Reading"=2.86038e-06}, {5.48124e-05, "Field Reading"=2.84027e-06}, {5.23329e-05, "Field Reading"=2.8203e-06}, {5.50509e-05, "Field Reading"=2.8003e-06}, {5.13792e-05, "Field Reading"=2.78033e-06}, {5.10931e-05, "Field Reading"=2.76037e-06}, {5.09977e-05, "Field Reading"=2.74024e-06}, {5.0211e-05, "Field Reading"=2.72026e-06}, {5.12838e-05, "Field Reading"=2.70028e-06}, {5.13792e-05, "Field Reading"=2.68032e-06}, {5.25713e-05, "Field Reading"=2.66034e-06}, {5.08785e-05, "Field Reading"=2.64038e-06}, {5.095e-05, "Field Reading"=2.62021e-06}, {5.03063e-05, "Field Reading"=2.60025e-06}, {4.94957e-05, "Field Reading"=2.58029e-06}, {5.04017e-05, "Field Reading"=2.56031e-06}, {4.99964e-05, "Field Reading"=2.54035e-06}, {4.89235e-05, "Field Reading"=2.52021e-06}, {5.04017e-05, "Field Reading"=2.50024e-06}, {5.10216e-05, "Field Reading"=2.48025e-06}, {5.28336e-05, "Field Reading"=2.46026e-06}, {5.06401e-05, "Field Reading"=2.44029e-06}, {4.96149e-05, "Field Reading"=2.42032e-06}, {4.9758e-05, "Field Reading"=2.40018e-06}, {4.8399e-05, "Field Reading"=2.38021e-06}, {4.91858e-05, "Field Reading"=2.36022e-06}, {4.92811e-05, "Field Reading"=2.34026e-06}, {5.00441e-05, "Field Reading"=2.32029e-06}, {5.03302e-05, "Field Reading"=2.30016e-06}, {4.67062e-05, "Field Reading"=2.28018e-06}, {4.73261e-05, "Field Reading"=2.2602e-06}, {4.62055e-05, "Field Reading"=2.24025e-06}, {4.76599e-05, "Field Reading"=2.22028e-06}, {4.59194e-05, "Field Reading"=2.20031e-06}, {4.51803e-05, "Field Reading"=2.18016e-06}, {4.64678e-05, "Field Reading"=2.16019e-06}, {4.673e-05, "Field Reading"=2.14022e-06}, {4.52995e-05, "Field Reading"=2.12023e-06}, {4.673e-05, "Field Reading"=2.10026e-06}, {4.49896e-05, "Field Reading"=2.08016e-06}, {4.52757e-05, "Field Reading"=2.06018e-06}, {4.60148e-05, "Field Reading"=2.0402e-06}, {4.68969e-05, "Field Reading"=2.02022e-06}, {4.84943e-05, "Field Reading"=2.00026e-06}, {4.60863e-05, "Field Reading"=1.98029e-06}, {4.55618e-05, "Field Reading"=1.96017e-06}, {4.59909e-05, "Field Reading"=1.9402e-06}, {4.56095e-05, "Field Reading"=1.92023e-06}, {3.34024e-05, "Field Reading"=1.90027e-06}, {3.438e-05, "Field Reading"=1.88029e-06}, {3.49998e-05, "Field Reading"=1.86015e-06}, {3.31879e-05, "Field Reading"=1.84018e-06}, {3.29494e-05, "Field Reading"=1.82021e-06}, {3.37124e-05, "Field Reading"=1.80025e-06}, {3.44992e-05, "Field Reading"=1.78026e-06}, {3.40462e-05, "Field Reading"=1.76028e-06}, {3.38316e-05, "Field Reading"=1.74015e-06}, {3.53336e-05, "Field Reading"=1.72018e-06}, {3.1209e-05, "Field Reading"=1.7002e-06}, {3.32594e-05, "Field Reading"=1.68023e-06}, {3.05176e-05, "Field Reading"=1.66025e-06}, {3.03984e-05, "Field Reading"=1.64011e-06}, {3.16143e-05, "Field Reading"=1.62014e-06}, {3.10659e-05, "Field Reading"=1.60016e-06}, {3.24965e-05, "Field Reading"=1.5802e-06}, {3.15666e-05, "Field Reading"=1.56021e-06}, {3.24488e-05, "Field Reading"=1.54025e-06}, {3.19719e-05, "Field Reading"=1.52011e-06}, {3.26633e-05, "Field Reading"=1.50013e-06}, {3.19958e-05, "Field Reading"=1.48016e-06}, {3.34263e-05, "Field Reading"=1.4602e-06}, {3.2258e-05, "Field Reading"=1.44021e-06}, {3.29494e-05, "Field Reading"=1.42007e-06}, {3.09467e-05, "Field Reading"=1.4001e-06}, {3.32117e-05, "Field Reading"=1.38013e-06}, {3.47137e-05, "Field Reading"=1.36016e-06}, {3.54528e-05, "Field Reading"=1.34019e-06}, {3.25203e-05, "Field Reading"=1.32023e-06}, {3.37124e-05, "Field Reading"=1.30008e-06}, {3.00646e-05, "Field Reading"=1.28011e-06}, {3.00884e-05, "Field Reading"=1.26011e-06}, {3.34024e-05, "Field Reading"=1.24014e-06}, {3.08275e-05, "Field Reading"=1.22018e-06}, {3.39746e-05, "Field Reading"=1.20004e-06}, {3.14474e-05, "Field Reading"=1.18007e-06}, {3.22819e-05, "Field Reading"=1.16009e-06}, {3.22819e-05, "Field Reading"=1.14014e-06}, {3.08514e-05, "Field Reading"=1.12016e-06}, {3.20435e-05, "Field Reading"=1.10017e-06}, {3.16858e-05, "Field Reading"=1.08002e-06}, {3.16858e-05, "Field Reading"=1.06006e-06}, {3.31163e-05, "Field Reading"=1.04009e-06}, {3.18766e-05, "Field Reading"=1.02015e-06}, {3.08514e-05, "Field Reading"=1.00012e-06}, {3.22342e-05, "Field Reading"=9.80119e-07}, {3.33548e-05, "Field Reading"=9.60115e-07}, {3.13759e-05, "Field Reading"=9.40125e-07}, {3.25918e-05, "Field Reading"=9.20117e-07}, {3.07798e-05, "Field Reading"=9.0013e-07}, {3.3474e-05, "Field Reading"=8.80123e-07}, {3.31402e-05, "Field Reading"=8.6013e-07}, {3.25441e-05, "Field Reading"=8.40122e-07}, {3.39746e-05, "Field Reading"=8.20114e-07}, {3.42607e-05, "Field Reading"=8.00128e-07}, {3.19719e-05, "Field Reading"=7.80116e-07}, {3.1352e-05, "Field Reading"=7.60129e-07}, {3.17335e-05, "Field Reading"=7.40128e-07}, {3.07798e-05, "Field Reading"=7.20136e-07}, {3.14951e-05, "Field Reading"=7.00131e-07}, {3.40462e-05, "Field Reading"=6.80142e-07}, {3.27826e-05, "Field Reading"=6.60129e-07}, {3.39985e-05, "Field Reading"=6.40121e-07}, {3.46422e-05, "Field Reading"=6.20128e-07}, {3.2568e-05, "Field Reading"=6.00115e-07}, {3.45469e-05, "Field Reading"=5.80128e-07}, {3.15905e-05, "Field Reading"=5.60114e-07}, {3.15666e-05, "Field Reading"=5.40122e-07}, {3.2115e-05, "Field Reading"=5.2011e-07}, {3.16381e-05, "Field Reading"=5.00119e-07}, {3.10898e-05, "Field Reading"=4.80109e-07}, {3.14951e-05, "Field Reading"=4.60099e-07}, {3.11613e-05, "Field Reading"=4.40104e-07}, {3.31163e-05, "Field Reading"=4.20101e-07}, {3.14951e-05, "Field Reading"=4.00103e-07}, {3.2711e-05, "Field Reading"=3.80089e-07}, {3.16858e-05, "Field Reading"=3.60101e-07}, {3.21388e-05, "Field Reading"=3.40087e-07}, {3.12328e-05, "Field Reading"=3.20073e-07}, {2.98738e-05, "Field Reading"=3.00087e-07}, {3.09944e-05, "Field Reading"=2.80073e-07}, {2.94447e-05, "Field Reading"=2.60077e-07}, {2.99931e-05, "Field Reading"=2.4007e-07}, {3.13997e-05, "Field Reading"=2.20077e-07}, {3.26395e-05, "Field Reading"=2.00066e-07}, {3.34263e-05, "Field Reading"=1.80071e-07}, {3.40939e-05, "Field Reading"=1.60062e-07}, {3.02553e-05, "Field Reading"=1.4005e-07}, {3.1805e-05, "Field Reading"=1.20057e-07}, {3.27349e-05, "Field Reading"=1.00008e-07}, {3.21627e-05, "Field Reading"=8.0008e-08}, {3.35932e-05, "Field Reading"=6.00067e-08}, {3.37124e-05, "Field Reading"=4.00059e-08}, {3.30925e-05, "Field Reading"=2.00026e-08}, {3.36409e-05, "Field Reading"=7.51019e-13}, {3.30687e-05, "Field Reading"=-1.99969e-08}, {3.56913e-05, "Field Reading"=-3.99991e-08}, {3.51429e-05, "Field Reading"=-6.00007e-08}, {3.39746e-05, "Field Reading"=-8.0001e-08}, {3.44992e-05, "Field Reading"=-9.99984e-08}, {3.33309e-05, "Field Reading"=-1.19949e-07}, {3.34978e-05, "Field Reading"=-1.39943e-07}, {3.21627e-05, "Field Reading"=-1.59942e-07}, {3.438e-05, "Field Reading"=-1.79956e-07}, {3.39031e-05, "Field Reading"=-1.99959e-07}, {3.50475e-05, "Field Reading"=-2.19972e-07}, {3.47137e-05, "Field Reading"=-2.39969e-07}, {3.48568e-05, "Field Reading"=-2.59962e-07}, {3.56197e-05, "Field Reading"=-2.79974e-07}, {3.52859e-05, "Field Reading"=-2.99967e-07}, {3.50475e-05, "Field Reading"=-3.19958e-07}, {3.65019e-05, "Field Reading"=-3.39971e-07}, {3.41654e-05, "Field Reading"=-3.59972e-07}, {3.38554e-05, "Field Reading"=-3.79981e-07}, {3.38316e-05, "Field Reading"=-3.99979e-07}, {3.44276e-05, "Field Reading"=-4.19974e-07}, {3.51906e-05, "Field Reading"=-4.39988e-07}, {3.57866e-05, "Field Reading"=-4.59982e-07}, {3.44992e-05, "Field Reading"=-4.79975e-07}, {3.51667e-05, "Field Reading"=-4.99986e-07}, {3.61443e-05, "Field Reading"=-5.19981e-07}, {3.47376e-05, "Field Reading"=-5.39992e-07}, {3.52383e-05, "Field Reading"=-5.59986e-07}, {3.44753e-05, "Field Reading"=-5.79987e-07}, {3.36885e-05, "Field Reading"=-6.00002e-07}, {3.56436e-05, "Field Reading"=-6.19996e-07}, {3.74079e-05, "Field Reading"=-6.39987e-07}, {3.49522e-05, "Field Reading"=-6.60002e-07}, {3.49045e-05, "Field Reading"=-6.79995e-07}, {3.48091e-05, "Field Reading"=-6.99983e-07}, {3.5882e-05, "Field Reading"=-7.19997e-07}, {3.52621e-05, "Field Reading"=-7.39992e-07}, {3.55959e-05, "Field Reading"=-7.6e-07}, {3.7384e-05, "Field Reading"=-7.79988e-07}, {3.42846e-05, "Field Reading"=-7.99982e-07}, {3.64065e-05, "Field Reading"=-8.19991e-07}, {3.438e-05, "Field Reading"=-8.39985e-07}, {3.54528e-05, "Field Reading"=-8.59976e-07}, {3.54052e-05, "Field Reading"=-8.7999e-07}, {3.77178e-05, "Field Reading"=-8.99985e-07}, {3.50237e-05, "Field Reading"=-9.19988e-07}, {3.33786e-05, "Field Reading"=-9.39984e-07}, {3.56913e-05, "Field Reading"=-9.59974e-07}, {3.55482e-05, "Field Reading"=-9.79982e-07}, {3.39985e-05, "Field Reading"=-9.99972e-07}, {3.51906e-05, "Field Reading"=-1.01998e-06}, {3.37362e-05, "Field Reading"=-1.03995e-06}, {3.35932e-05, "Field Reading"=-1.05992e-06}, {3.38316e-05, "Field Reading"=-1.07989e-06}, {3.48091e-05, "Field Reading"=-1.09986e-06}, {3.63112e-05, "Field Reading"=-1.11985e-06}, {3.67641e-05, "Field Reading"=-1.14001e-06}, {3.53813e-05, "Field Reading"=-1.15998e-06}, {3.28779e-05, "Field Reading"=-1.17996e-06}, {3.55244e-05, "Field Reading"=-1.19994e-06}, {3.31163e-05, "Field Reading"=-1.21992e-06}, {3.23296e-05, "Field Reading"=-1.23988e-06}, {3.39746e-05, "Field Reading"=-1.25986e-06}, {3.29971e-05, "Field Reading"=-1.28001e-06}, {3.39508e-05, "Field Reading"=-1.29998e-06}, {3.35217e-05, "Field Reading"=-1.31997e-06}, {3.19242e-05, "Field Reading"=-1.33995e-06}, {3.36885e-05, "Field Reading"=-1.35992e-06}, {3.35932e-05, "Field Reading"=-1.37988e-06}, {3.17097e-05, "Field Reading"=-1.40001e-06}, {3.22104e-05, "Field Reading"=-1.41998e-06}, {3.02315e-05, "Field Reading"=-1.43997e-06}, {3.11852e-05, "Field Reading"=-1.45997e-06}, {2.92301e-05, "Field Reading"=-1.47993e-06}, {3.04937e-05, "Field Reading"=-1.4999e-06}, {3.19481e-05, "Field Reading"=-1.52004e-06}, {3.29494e-05, "Field Reading"=-1.53999e-06}, {3.30448e-05, "Field Reading"=-1.55997e-06}, {3.14713e-05, "Field Reading"=-1.57995e-06}, {3.20911e-05, "Field Reading"=-1.59992e-06}, {3.2115e-05, "Field Reading"=-1.61993e-06}, {3.00646e-05, "Field Reading"=-1.6399e-06}, {3.22342e-05, "Field Reading"=-1.66003e-06}, {3.2568e-05, "Field Reading"=-1.68e-06}, {3.14713e-05, "Field Reading"=-1.69998e-06}, {3.28064e-05, "Field Reading"=-1.71996e-06}, {3.39985e-05, "Field Reading"=-1.73994e-06}, {3.46899e-05, "Field Reading"=-1.75992e-06}, {3.34024e-05, "Field Reading"=-1.78007e-06}, {2.76566e-05, "Field Reading"=-1.80008e-06}, {3.20911e-05, "Field Reading"=-1.82006e-06}, {3.29971e-05, "Field Reading"=-1.83999e-06}, {3.36885e-05, "Field Reading"=-1.85996e-06}, {3.25918e-05, "Field Reading"=-1.87994e-06}, {3.3474e-05, "Field Reading"=-1.90008e-06}, {3.34024e-05, "Field Reading"=-1.92007e-06}, {3.438e-05, "Field Reading"=-1.94004e-06}, {3.38078e-05, "Field Reading"=-1.96002e-06}, {3.35932e-05, "Field Reading"=-1.97999e-06}, {3.2711e-05, "Field Reading"=-1.99996e-06}, {3.15666e-05, "Field Reading"=-2.01994e-06}, {3.15189e-05, "Field Reading"=-2.04008e-06}, {3.27349e-05, "Field Reading"=-2.06006e-06}, {3.23534e-05, "Field Reading"=-2.08004e-06}, {3.40462e-05, "Field Reading"=-2.1e-06}, {3.46899e-05, "Field Reading"=-2.11998e-06}, {3.5429e-05, "Field Reading"=-2.13997e-06}, {3.49998e-05, "Field Reading"=-2.16011e-06}, {3.52144e-05, "Field Reading"=-2.18008e-06}, {3.41892e-05, "Field Reading"=-2.20005e-06}, {3.50475e-05, "Field Reading"=-2.22002e-06}, {3.47853e-05, "Field Reading"=-2.24e-06}, {3.33071e-05, "Field Reading"=-2.25997e-06}, {3.40462e-05, "Field Reading"=-2.28013e-06}, {3.47614e-05, "Field Reading"=-2.30012e-06}, {3.35455e-05, "Field Reading"=-2.32008e-06}, {3.55959e-05, "Field Reading"=-2.34003e-06}, {3.56674e-05, "Field Reading"=-2.36003e-06}, {3.48568e-05, "Field Reading"=-2.38002e-06}, {3.65496e-05, "Field Reading"=-2.39997e-06}, {3.55244e-05, "Field Reading"=-2.42011e-06}, {3.42131e-05, "Field Reading"=-2.44008e-06}, {3.30687e-05, "Field Reading"=-2.46005e-06}, {3.48091e-05, "Field Reading"=-2.48005e-06}, {3.16381e-05, "Field Reading"=-2.50002e-06}, {3.34024e-05, "Field Reading"=-2.52e-06}, {3.47614e-05, "Field Reading"=-2.54015e-06}, {3.29018e-05, "Field Reading"=-2.56012e-06}, {3.51906e-05, "Field Reading"=-2.58008e-06}, {3.57389e-05, "Field Reading"=-2.60006e-06}, {3.43323e-05, "Field Reading"=-2.62004e-06}, {3.22104e-05, "Field Reading"=-2.64004e-06}, {3.15905e-05, "Field Reading"=-2.66018e-06}, {3.26633e-05, "Field Reading"=-2.68014e-06}, {3.21388e-05, "Field Reading"=-2.70013e-06}, {1.4472e-05, "Field Reading"=-2.72009e-06}, {1.52588e-05, "Field Reading"=-2.74005e-06}, {1.4925e-05, "Field Reading"=-2.76003e-06}, {1.44243e-05, "Field Reading"=-2.78001e-06}, {1.4329e-05, "Field Reading"=-2.80015e-06}, {1.49727e-05, "Field Reading"=-2.82015e-06}, {1.19925e-05, "Field Reading"=-2.84013e-06}, {1.02758e-05, "Field Reading"=-2.86011e-06}, {1.20401e-05, "Field Reading"=-2.88007e-06}, {1.14918e-05, "Field Reading"=-2.90005e-06}, {1.1301e-05, "Field Reading"=-2.92019e-06}, {1.15871e-05, "Field Reading"=-2.94017e-06}, {1.33038e-05, "Field Reading"=-2.96015e-06}, {1.1611e-05, "Field Reading"=-2.98015e-06}, {9.91821e-06, "Field Reading"=-3.00013e-06}, {9.29832e-06, "Field Reading"=-3.02008e-06}, {9.91821e-06, "Field Reading"=-3.04023e-06}, {1.05858e-05, "Field Reading"=-3.0602e-06}, {1.06335e-05, "Field Reading"=-3.08018e-06}, {1.05143e-05, "Field Reading"=-3.10014e-06}, {1.04189e-05, "Field Reading"=-3.12011e-06}, {1.00613e-05, "Field Reading"=-3.14009e-06}, {1.01328e-05, "Field Reading"=-3.16009e-06}, {9.2268e-06, "Field Reading"=-3.18022e-06}, {9.72748e-06, "Field Reading"=-3.20019e-06}, {8.7738e-06, "Field Reading"=-3.22016e-06}, {1.0705e-05, "Field Reading"=-3.24013e-06}, {9.82285e-06, "Field Reading"=-3.26008e-06}, {1.10865e-05, "Field Reading"=-3.28005e-06}, {8.39233e-06, "Field Reading"=-3.3002e-06}, {9.13143e-06, "Field Reading"=-3.3202e-06}, {8.41618e-06, "Field Reading"=-3.34016e-06}, {1.01805e-05, "Field Reading"=-3.36014e-06}, {9.41753e-06, "Field Reading"=-3.3801e-06}, {7.77245e-06, "Field Reading"=-3.40008e-06}, {8.15392e-06, "Field Reading"=-3.42023e-06}, {8.63075e-06, "Field Reading"=-3.44019e-06}, {8.29697e-06, "Field Reading"=-3.46017e-06}, {9.36985e-06, "Field Reading"=-3.48014e-06}, {7.03335e-06, "Field Reading"=-3.50013e-06}, {5.6982e-06, "Field Reading"=-3.5201e-06}, {6.58035e-06, "Field Reading"=-3.54008e-06}, {6.8903e-06, "Field Reading"=-3.56023e-06}, {6.34193e-06, "Field Reading"=-3.58021e-06}, {8.08239e-06, "Field Reading"=-3.60018e-06}, {5.93662e-06, "Field Reading"=-3.62014e-06}, {6.91414e-06, "Field Reading"=-3.6401e-06}, {6.00815e-06, "Field Reading"=-3.66009e-06}, {5.76973e-06, "Field Reading"=-3.68023e-06}, {6.03199e-06, "Field Reading"=-3.70019e-06}, {8.44002e-06, "Field Reading"=-3.72017e-06}, {4.69685e-06, "Field Reading"=-3.74014e-06}, {6.67572e-06, "Field Reading"=-3.76013e-06}, {5.29289e-06, "Field Reading"=-3.78009e-06}, {5.10216e-06, "Field Reading"=-3.80023e-06}, {6.29425e-06, "Field Reading"=-3.8202e-06}, {5.67436e-06, "Field Reading"=-3.84019e-06}, {5.45979e-06, "Field Reading"=-3.86017e-06}, {4.41074e-06, "Field Reading"=-3.88016e-06}, {4.12464e-06, "Field Reading"=-3.90013e-06}, {2.00272e-06, "Field Reading"=-3.9201e-06}, {3.48091e-06, "Field Reading"=-3.94023e-06}, {3.09944e-06, "Field Reading"=-3.9602e-06}, {3.93391e-06, "Field Reading"=-3.98019e-06}, {4.86374e-06, "Field Reading"=-4.00018e-06}, {4.55379e-06, "Field Reading"=-4.02014e-06}, {3.71933e-06, "Field Reading"=-4.0401e-06}, {3.93391e-06, "Field Reading"=-4.06024e-06}, {-2.14577e-07, "Field Reading"=-4.08021e-06}, {2.86102e-06, "Field Reading"=-4.10016e-06}, {1.26362e-06, "Field Reading"=-4.12013e-06}, {1.64509e-06, "Field Reading"=-4.1401e-06}, {8.10623e-07, "Field Reading"=-4.16007e-06}, {1.28746e-06, "Field Reading"=-4.18024e-06}, {9.29832e-07, "Field Reading"=-4.20022e-06}, {-4.76837e-08, "Field Reading"=-4.22019e-06}, {-1.19209e-07, "Field Reading"=-4.24015e-06}, {3.33786e-07, "Field Reading"=-4.26012e-06}, {3.33786e-07, "Field Reading"=-4.2801e-06}, {-7.39098e-07, "Field Reading"=-4.30007e-06}, {-1.07288e-06, "Field Reading"=-4.32021e-06}, {9.53674e-08, "Field Reading"=-4.34021e-06}, {1.38283e-06, "Field Reading"=-4.36017e-06}, {6.67572e-07, "Field Reading"=-4.38014e-06}, {9.53674e-08, "Field Reading"=-4.40011e-06}, {-2.09808e-06, "Field Reading"=-4.42007e-06}, {-1.50204e-06, "Field Reading"=-4.44022e-06}, {0.0, "Field Reading"=-4.46019e-06}, {-2.45571e-06, "Field Reading"=-4.48017e-06}, {-4.91142e-06, "Field Reading"=-4.50014e-06}, {-2.86102e-06, "Field Reading"=-4.52016e-06}, {-2.45571e-06, "Field Reading"=-4.54011e-06}, {-3.14713e-06, "Field Reading"=-4.56025e-06}, {-4.3869e-06, "Field Reading"=-4.58023e-06}, {-3.3617e-06, "Field Reading"=-4.60019e-06}, {-4.48227e-06, "Field Reading"=-4.62018e-06}, {-1.14441e-06, "Field Reading"=-4.64016e-06}, {-3.88622e-06, "Field Reading"=-4.66012e-06}, {-3.43323e-06, "Field Reading"=-4.68009e-06}, {-5.17368e-06, "Field Reading"=-4.70024e-06}, {-4.14848e-06, "Field Reading"=-4.7202e-06}, {-4.81606e-06, "Field Reading"=-4.74018e-06}, {-5.03063e-06, "Field Reading"=-4.76016e-06}, {-5.79357e-06, "Field Reading"=-4.78014e-06}, {-3.24249e-06, "Field Reading"=-4.80012e-06}, {-5.81741e-06, "Field Reading"=-4.82026e-06}, {-5.38826e-06, "Field Reading"=-4.8402e-06}, {-4.91142e-06, "Field Reading"=-4.86021e-06}, {-6.48499e-06, "Field Reading"=-4.88018e-06}, {-4.69685e-06, "Field Reading"=-4.90016e-06}, {-7.53403e-06, "Field Reading"=-4.92013e-06}, {-6.4373e-06, "Field Reading"=-4.94029e-06}, {-6.98566e-06, "Field Reading"=-4.96024e-06}, {-7.10487e-06, "Field Reading"=-4.98021e-06}, {-9.05991e-06, "Field Reading"=-5.00019e-06}, {-7.89166e-06, "Field Reading"=-5.00018e-06}, {-6.8903e-06, "Field Reading"=-4.98022e-06}, {-7.7486e-06, "Field Reading"=-4.96024e-06}, {-5.79357e-06, "Field Reading"=-4.94027e-06}, {-5.98431e-06, "Field Reading"=-4.92013e-06}, {-5.26905e-06, "Field Reading"=-4.90015e-06}, {-6.31809e-06, "Field Reading"=-4.88018e-06}, {-5.74589e-06, "Field Reading"=-4.86022e-06}, {-4.74453e-06, "Field Reading"=-4.84022e-06}, {-4.79221e-06, "Field Reading"=-4.82023e-06}, {-7.98702e-06, "Field Reading"=-4.8001e-06}, {-5.53131e-06, "Field Reading"=-4.78013e-06}, {-6.03199e-06, "Field Reading"=-4.76014e-06}, {-6.34193e-06, "Field Reading"=-4.74017e-06}, {-4.95911e-06, "Field Reading"=-4.7202e-06}, {-6.98566e-06, "Field Reading"=-4.70023e-06}, {-4.1008e-06, "Field Reading"=-4.68007e-06}, {-5.07832e-06, "Field Reading"=-4.66011e-06}, {-5.76973e-06, "Field Reading"=-4.64014e-06}, {-4.48227e-06, "Field Reading"=-4.62017e-06}, {-2.26498e-06, "Field Reading"=-4.60021e-06}, {-2.67029e-06, "Field Reading"=-4.58025e-06}, {-4.05312e-07, "Field Reading"=-4.56028e-06}, {-2.6226e-06, "Field Reading"=-4.54015e-06}, {-1.07288e-06, "Field Reading"=-4.52017e-06}, {-2.98023e-06, "Field Reading"=-4.50018e-06}, {-1.33514e-06, "Field Reading"=-4.48022e-06}, {-2.7895e-06, "Field Reading"=-4.46025e-06}, {-2.24113e-06, "Field Reading"=-4.44027e-06}, {-2.19345e-06, "Field Reading"=-4.42013e-06}, {-1.85966e-06, "Field Reading"=-4.40015e-06}, {-3.88622e-06, "Field Reading"=-4.3802e-06}, {-3.98159e-06, "Field Reading"=-4.36022e-06}, {-1.85966e-06, "Field Reading"=-4.34024e-06}, {-2.16961e-06, "Field Reading"=-4.32025e-06}, {-2.59876e-06, "Field Reading"=-4.30011e-06}, {1.00136e-06, "Field Reading"=-4.28013e-06}, {-1.43051e-07, "Field Reading"=-4.26016e-06}, {-6.19888e-07, "Field Reading"=-4.24018e-06}, {-2.86102e-07, "Field Reading"=-4.22022e-06}, {-7.15256e-08, "Field Reading"=-4.20025e-06}, {-1.90735e-07, "Field Reading"=-4.18027e-06}, {2.02656e-06, "Field Reading"=-4.1601e-06}, {3.33786e-06, "Field Reading"=-4.14013e-06}, {2.67029e-06, "Field Reading"=-4.12015e-06}, {1.90735e-06, "Field Reading"=-4.10018e-06}, {2.81334e-06, "Field Reading"=-4.08022e-06}, {5.26905e-06, "Field Reading"=-4.06025e-06}, {2.24113e-06, "Field Reading"=-4.04012e-06}, {3.24249e-06, "Field Reading"=-4.02014e-06}, {1.81198e-06, "Field Reading"=-4.00017e-06}, {3.48091e-06, "Field Reading"=-3.98017e-06}, {5.55515e-06, "Field Reading"=-3.96021e-06}, {4.22001e-06, "Field Reading"=-3.94024e-06}, {3.95775e-06, "Field Reading"=-3.92011e-06}, {4.74453e-06, "Field Reading"=-3.90013e-06}, {5.74589e-06, "Field Reading"=-3.88016e-06}, {4.3869e-06, "Field Reading"=-3.86018e-06}, {3.86238e-06, "Field Reading"=-3.8402e-06}, {4.19617e-06, "Field Reading"=-3.8202e-06}, {3.21865e-06, "Field Reading"=-3.80023e-06}, {7.51019e-06, "Field Reading"=-3.78009e-06}, {3.50475e-06, "Field Reading"=-3.76013e-06}, {5.88894e-06, "Field Reading"=-3.74013e-06}, {3.86238e-06, "Field Reading"=-3.72017e-06}, {5.17368e-06, "Field Reading"=-3.70019e-06}, {4.79221e-06, "Field Reading"=-3.68023e-06}, {6.05583e-06, "Field Reading"=-3.66009e-06}, {6.12736e-06, "Field Reading"=-3.64009e-06}, {6.7234e-06, "Field Reading"=-3.62014e-06}, {7.55787e-06, "Field Reading"=-3.60018e-06}, {8.4877e-06, "Field Reading"=-3.58022e-06}, {7.96318e-06, "Field Reading"=-3.56022e-06}, {8.74996e-06, "Field Reading"=-3.54008e-06}, {8.86917e-06, "Field Reading"=-3.52009e-06}, {9.15527e-06, "Field Reading"=-3.50014e-06}, {7.29561e-06, "Field Reading"=-3.48014e-06}, {8.13007e-06, "Field Reading"=-3.46017e-06}, {9.34601e-06, "Field Reading"=-3.44021e-06}, {1.02043e-05, "Field Reading"=-3.42023e-06}, {8.98838e-06, "Field Reading"=-3.40008e-06}, {9.60827e-06, "Field Reading"=-3.3801e-06}, {9.70364e-06, "Field Reading"=-3.36012e-06}, {1.12057e-05, "Field Reading"=-3.34015e-06}, {1.02043e-05, "Field Reading"=-3.32018e-06}, {1.08719e-05, "Field Reading"=-3.30018e-06}, {8.51154e-06, "Field Reading"=-3.28004e-06}, {1.09196e-05, "Field Reading"=-3.26007e-06}, {1.11341e-05, "Field Reading"=-3.2401e-06}, {1.24693e-05, "Field Reading"=-3.22015e-06}, {1.21355e-05, "Field Reading"=-3.20016e-06}, {1.2064e-05, "Field Reading"=-3.18019e-06}, {1.32561e-05, "Field Reading"=-3.16004e-06}, {1.21117e-05, "Field Reading"=-3.14004e-06}, {1.41859e-05, "Field Reading"=-3.12007e-06}, {1.42574e-05, "Field Reading"=-3.10009e-06}, {1.31607e-05, "Field Reading"=-3.08011e-06}, {1.42097e-05, "Field Reading"=-3.06013e-06}, {1.49488e-05, "Field Reading"=-3.04016e-06}, {1.39713e-05, "Field Reading"=-3.02004e-06}, {1.41859e-05, "Field Reading"=-3.00007e-06}, {1.34945e-05, "Field Reading"=-2.9801e-06}, {1.33514e-05, "Field Reading"=-2.96012e-06}, {1.23024e-05, "Field Reading"=-2.94013e-06}, {1.33753e-05, "Field Reading"=-2.92015e-06}, {1.56879e-05, "Field Reading"=-2.90002e-06}, {1.28746e-05, "Field Reading"=-2.88004e-06}, {1.66178e-05, "Field Reading"=-2.86007e-06}, {1.31369e-05, "Field Reading"=-2.8401e-06}, {1.53542e-05, "Field Reading"=-2.82012e-06}, {1.56641e-05, "Field Reading"=-2.80012e-06}, {1.72138e-05, "Field Reading"=-2.77999e-06}, {1.8096e-05, "Field Reading"=-2.76002e-06}, {1.89543e-05, "Field Reading"=-2.74005e-06}, {1.688e-05, "Field Reading"=-2.72008e-06}, {1.719e-05, "Field Reading"=-2.7001e-06}, {1.61409e-05, "Field Reading"=-2.68015e-06}, {1.88589e-05, "Field Reading"=-2.66018e-06}, {1.76191e-05, "Field Reading"=-2.64004e-06}, {1.85728e-05, "Field Reading"=-2.62004e-06}, {1.73092e-05, "Field Reading"=-2.60007e-06}, {1.92404e-05, "Field Reading"=-2.5801e-06}, {1.94788e-05, "Field Reading"=-2.56012e-06}, {1.81675e-05, "Field Reading"=-2.54015e-06}, {1.77622e-05, "Field Reading"=-2.52001e-06}, {1.63078e-05, "Field Reading"=-2.50002e-06}, {1.85251e-05, "Field Reading"=-2.48006e-06}, {2.05755e-05, "Field Reading"=-2.46005e-06}, {1.90973e-05, "Field Reading"=-2.44007e-06}, {1.96695e-05, "Field Reading"=-2.42012e-06}, {1.95503e-05, "Field Reading"=-2.39999e-06}, {1.82152e-05, "Field Reading"=-2.38002e-06}, {1.94073e-05, "Field Reading"=-2.36004e-06}, {2.04802e-05, "Field Reading"=-2.34005e-06}, {2.02656e-05, "Field Reading"=-2.32008e-06}, {2.04086e-05, "Field Reading"=-2.30011e-06}, {2.05278e-05, "Field Reading"=-2.28012e-06}, {2.17438e-05, "Field Reading"=-2.26e-06}, {2.10285e-05, "Field Reading"=-2.24003e-06}, {2.12193e-05, "Field Reading"=-2.22004e-06}, {2.26974e-05, "Field Reading"=-2.20006e-06}, {2.19584e-05, "Field Reading"=-2.18009e-06}, {2.29597e-05, "Field Reading"=-2.1601e-06}, {2.43902e-05, "Field Reading"=-2.13998e-06}, {2.41756e-05, "Field Reading"=-2.11997e-06}, {2.35796e-05, "Field Reading"=-2.1e-06}, {2.57254e-05, "Field Reading"=-2.08004e-06}, {2.34127e-05, "Field Reading"=-2.06009e-06}, {2.36988e-05, "Field Reading"=-2.04011e-06}, {2.18391e-05, "Field Reading"=-2.01996e-06}, {2.4724e-05, "Field Reading"=-1.99999e-06}, {2.50578e-05, "Field Reading"=-1.98002e-06}, {2.49624e-05, "Field Reading"=-1.96007e-06}, {2.43902e-05, "Field Reading"=-1.94008e-06}, {3.61204e-05, "Field Reading"=-1.92011e-06}, {3.75986e-05, "Field Reading"=-1.90012e-06}, {3.59297e-05, "Field Reading"=-1.87998e-06}, {3.57628e-05, "Field Reading"=-1.86e-06}, {3.53575e-05, "Field Reading"=-1.84001e-06}, {3.4523e-05, "Field Reading"=-1.82007e-06}, {3.44992e-05, "Field Reading"=-1.80008e-06}, {3.36885e-05, "Field Reading"=-1.7801e-06}, {3.43084e-05, "Field Reading"=-1.75993e-06}, {3.75509e-05, "Field Reading"=-1.73996e-06}, {3.59058e-05, "Field Reading"=-1.71997e-06}, {3.36647e-05, "Field Reading"=-1.70002e-06}, {3.42846e-05, "Field Reading"=-1.68003e-06}, {3.30687e-05, "Field Reading"=-1.66005e-06}, {3.407e-05, "Field Reading"=-1.63991e-06}, {3.37601e-05, "Field Reading"=-1.61995e-06}, {3.55005e-05, "Field Reading"=-1.59993e-06}, {3.25203e-05, "Field Reading"=-1.57996e-06}, {3.39031e-05, "Field Reading"=-1.55997e-06}, {3.35217e-05, "Field Reading"=-1.53999e-06}, {3.35932e-05, "Field Reading"=-1.52001e-06}, {3.2711e-05, "Field Reading"=-1.49987e-06}, {3.6025e-05, "Field Reading"=-1.4799e-06}, {3.37601e-05, "Field Reading"=-1.45993e-06}, {3.32594e-05, "Field Reading"=-1.43991e-06}, {3.53336e-05, "Field Reading"=-1.41995e-06}, {3.4523e-05, "Field Reading"=-1.39997e-06}, {3.52859e-05, "Field Reading"=-1.37983e-06}, {3.50952e-05, "Field Reading"=-1.35987e-06}, {3.55721e-05, "Field Reading"=-1.3399e-06}, {3.5429e-05, "Field Reading"=-1.31994e-06}, {3.37362e-05, "Field Reading"=-1.29997e-06}, {3.41654e-05, "Field Reading"=-1.27999e-06}, {3.30448e-05, "Field Reading"=-1.25983e-06}, {3.30925e-05, "Field Reading"=-1.23984e-06}, {3.16143e-05, "Field Reading"=-1.21987e-06}, {3.28064e-05, "Field Reading"=-1.19991e-06}, {3.29971e-05, "Field Reading"=-1.17993e-06}, {3.32117e-05, "Field Reading"=-1.15996e-06}, {3.21388e-05, "Field Reading"=-1.13999e-06}, {3.49283e-05, "Field Reading"=-1.11983e-06}, {3.39985e-05, "Field Reading"=-1.09984e-06}, {3.04937e-05, "Field Reading"=-1.07987e-06}, {3.1805e-05, "Field Reading"=-1.0599e-06}, {3.36885e-05, "Field Reading"=-1.03994e-06}, {3.3617e-05, "Field Reading"=-1.01997e-06}, {3.42846e-05, "Field Reading"=-9.99967e-07}, {3.46899e-05, "Field Reading"=-9.79982e-07}, {3.51191e-05, "Field Reading"=-9.59967e-07}, {3.44992e-05, "Field Reading"=-9.39973e-07}, {3.46661e-05, "Field Reading"=-9.19983e-07}, {3.6335e-05, "Field Reading"=-8.99972e-07}, {3.36885e-05, "Field Reading"=-8.79985e-07}, {3.46184e-05, "Field Reading"=-8.59972e-07}, {3.49045e-05, "Field Reading"=-8.39981e-07}, {3.55482e-05, "Field Reading"=-8.1999e-07}, {3.29018e-05, "Field Reading"=-7.9998e-07}, {3.45945e-05, "Field Reading"=-7.79988e-07}, {3.45469e-05, "Field Reading"=-7.59993e-07}, {3.56436e-05, "Field Reading"=-7.39992e-07}, {3.27587e-05, "Field Reading"=-7.19995e-07}, {3.49998e-05, "Field Reading"=-6.99987e-07}, {3.54052e-05, "Field Reading"=-6.79995e-07}, {3.6335e-05, "Field Reading"=-6.6e-07}, {3.407e-05, "Field Reading"=-6.39983e-07}, {3.37362e-05, "Field Reading"=-6.19994e-07}, {3.36885e-05, "Field Reading"=-6.00001e-07}, {3.26395e-05, "Field Reading"=-5.79989e-07}, {3.54767e-05, "Field Reading"=-5.5999e-07}, {3.23057e-05, "Field Reading"=-5.39999e-07}, {3.2258e-05, "Field Reading"=-5.19986e-07}, {3.26872e-05, "Field Reading"=-4.99998e-07}, {3.21627e-05, "Field Reading"=-4.79984e-07}, {3.10183e-05, "Field Reading"=-4.59985e-07}, {3.33548e-05, "Field Reading"=-4.39989e-07}, {3.14236e-05, "Field Reading"=-4.19979e-07}, {3.19481e-05, "Field Reading"=-3.99979e-07}, {3.21627e-05, "Field Reading"=-3.79983e-07}, {3.04222e-05, "Field Reading"=-3.5997e-07}, {3.19958e-05, "Field Reading"=-3.39973e-07}, {3.24965e-05, "Field Reading"=-3.1996e-07}, {3.28541e-05, "Field Reading"=-2.99963e-07}, {3.1805e-05, "Field Reading"=-2.79968e-07}, {3.03268e-05, "Field Reading"=-2.59957e-07}, {2.97546e-05, "Field Reading"=-2.39959e-07}, {3.1662e-05, "Field Reading"=-2.19962e-07}, {3.09467e-05, "Field Reading"=-1.99949e-07}, {3.01123e-05, "Field Reading"=-1.7995e-07}, {3.03984e-05, "Field Reading"=-1.59933e-07}, {3.24249e-05, "Field Reading"=-1.39938e-07}, {3.14474e-05, "Field Reading"=-1.19943e-07}, {2.95639e-05, "Field Reading"=-9.99978e-08}, {3.02553e-05, "Field Reading"=-8.00006e-08}, {3.19958e-05, "Field Reading"=-6.00005e-08}, {3.08275e-05, "Field Reading"=-3.99989e-08}, {3.16381e-05, "Field Reading"=-1.99967e-08}, {2.89917e-05, "Field Reading"=4.3869e-12}]
  out "data":dbl[](array[numeric])=[2.89917e-05, 4.3869e-12, 6608698.625453053]
  in  "Source meter K2636B":refnum<visa-resource-name>="GPIB0::26::INSTR"
  in  "Step":dbl[](array[numeric])=[2e-08, 2e-08, 2e-08] min=-3000.0 max=3000.0 format="%.1e"
  in  "To":dbl[](array[numeric])=[5e-06, -5e-06, 0.0] min=-3000.0 max=3000.0 format="%.1e"
  in  "From":dbl[](array[numeric])=[0.0, 5e-06, -5e-06] min=-3000.0 max=3000.0 format="%.1e"
  in  "file name":string="045_29-10-2022_002_DevD2_I_39-36_V_42-41_DC_IV_ZF_baseT_K2636B"
  out "File path":path=path "D:/Pranava/Data/PtTe2/29-10-2022/002/045_29-10-2022_002_DevD2_I_39-36_V_42-41_DC_IV_ZF_baseT_K2636B.dat"
  # ".dat"
  # "2-point sense"
  # "Set Current (A)"
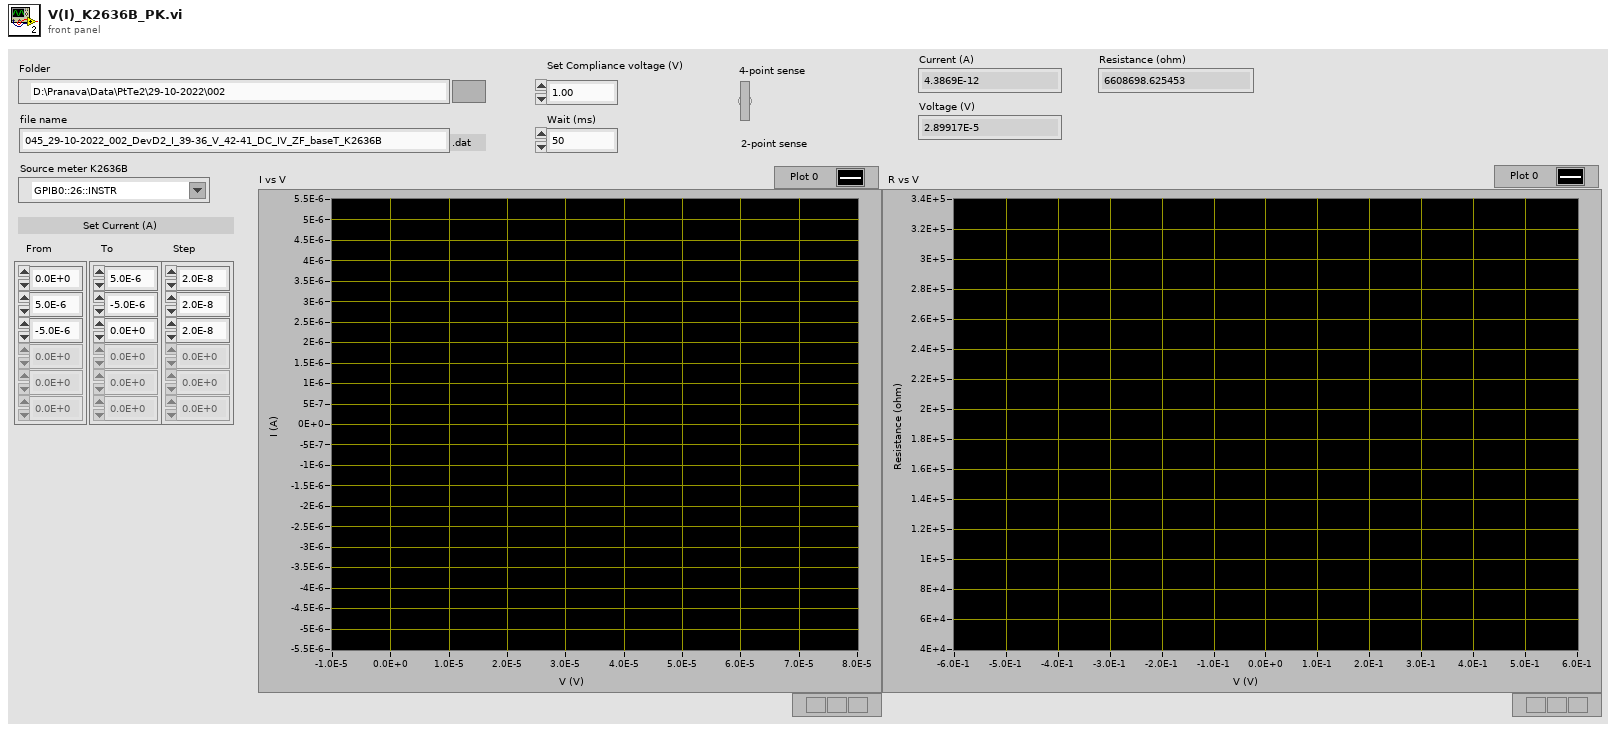
[diagram p1: front panel]
types:
  T1 = enum16{"open", "replace", "create", "open or create", "replace or create", "replace or create with confirmation"}
  T2 = cluster{"Last Voltage (V)":dbl, "Last Current (A)":dbl}
  T3 = cluster{"Last Voltage (V)":dbl, "Last Current (A)":dbl}[]
  T4 = cluster{"Last Voltage (V)":dbl, "Field Reading":dbl}[]
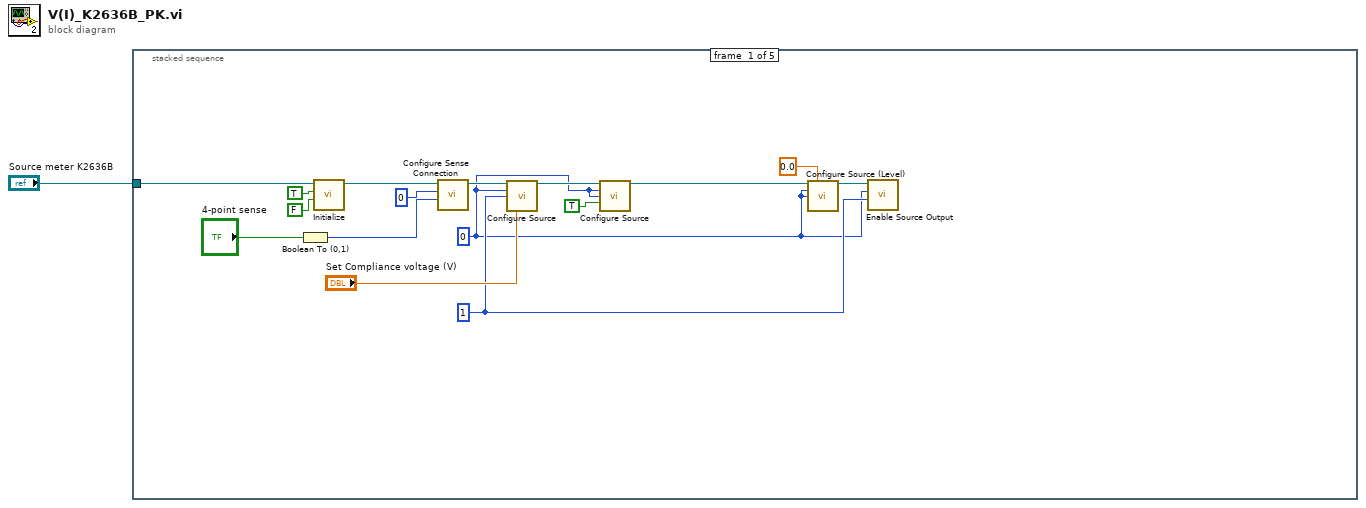
[diagram p0: block diagram]
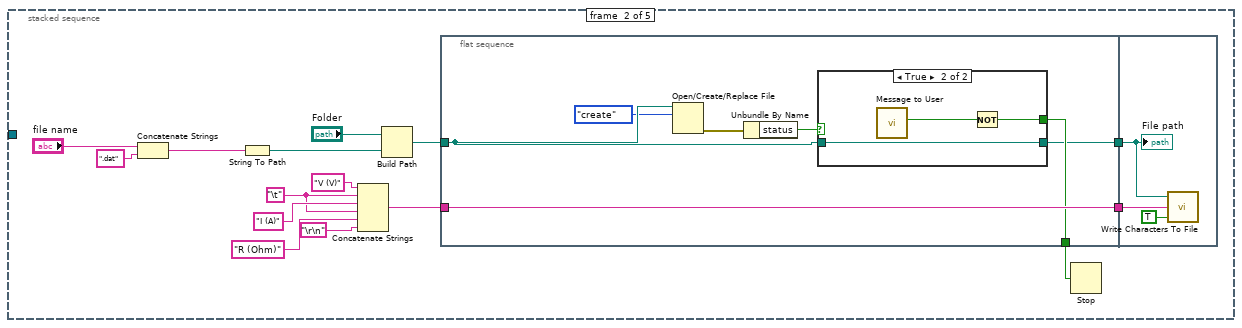
[diagram p2: hidden frame]
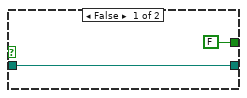
[diagram p3: hidden frame]
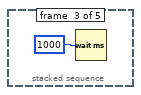
[diagram p4: hidden frame]
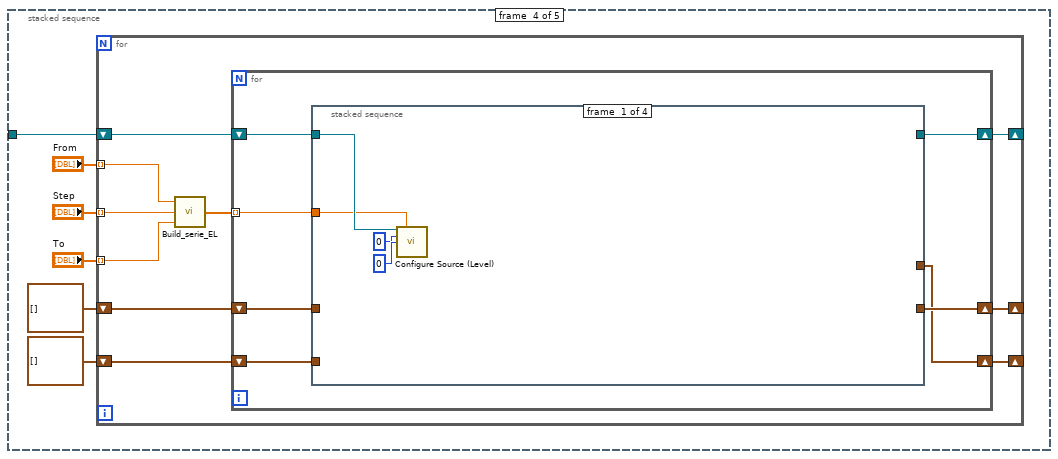
[diagram p5: hidden frame]
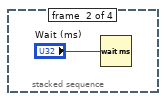
[diagram p6: hidden frame]
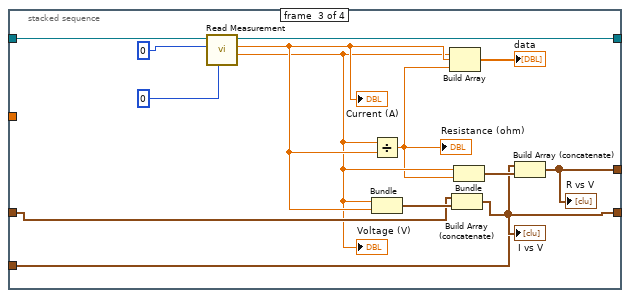
[diagram p7: hidden frame]
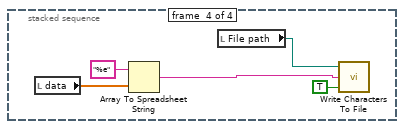
[diagram p8: hidden frame]
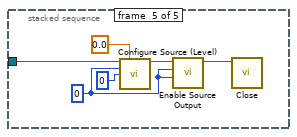
[diagram p9: hidden frame]
diagram:
  n1 = stacked-sequence {
    tunnel: "Source meter K2636B" -> [w17 _ _ w51 w100]
    frame #0 {
      w3 = 0
      w5 = 1
      n2 = Boolean To (0,1)(Boolean="4-point sense") -> (0, 1=w7:i16)
      n3 = call "Initialize.vi"("Reset (True)"=FALSE, "ID Query (True)"=TRUE, "VISA resource name"=w17) -> ("VISA resource name out"=w11:refnum<visa-resource-name>)  [unwired: 7 in, 1 out]
      n4 = call "Configure Sense Connection.vi"("Sense Mode (0: Local Sense)"=w7, "Source Measure Unit Channel (0: Channel A)"=0, "VISA resource name"=w11) -> ("VISA resource name out"=w10:refnum<visa-resource-name>)  [unwired: 7 in, 1 out]
      n5 = call-poly "Configure Source.vi"("VISA resource name"=w10, "Source Measure Unit Channel (0: Channel A)"=w3, "Limit Type (1: Voltage)"=w5, "Voltage Limit (20 V)"="Set Compliance voltage (V)") -> ("VISA resource name out"=w16:refnum<visa-resource-name>)  [unwired: 10 in, 1 out]
      n6 = call-poly "Configure Source.vi"("VISA resource name"=w16, "Source Measure Unit Channel (0: Channel A)"=w3, "Range Type (1: Voltage)"=w3, "Auto Range (T: Enable)"=TRUE) -> ("VISA resource name out"=w15:refnum<visa-resource-name>)  [unwired: 10 in, 1 out]
      n7 = call "Configure Source (Level).vi"("VISA resource name"=w15, "Current Level (0 A)"=0.0, "Source Measure Unit Channel (0: Channel A)"=w3, "Level Type (1: Voltage)"=w3) -> ("VISA resource name out"=w14:refnum<visa-resource-name>)  [unwired: 10 in, 1 out]
      n8 = call "Enable Source Output.vi"("Output Mode (0: Turn off)"=w5, "Source Measure Unit Channel (0: Channel A)"=w3, "VISA resource name"=w14) -> ()  [unwired: 7 in, 2 out]
    }
    frame #1 {
      w23 = "\t"
      n9 = Concatenate Strings("file name", ".dat" ("string")) -> (w29:string)
      n10 = String To Path(string=w29) -> (path=w19:path)
      n11 = Concatenate Strings("V (V)" ("string"), w23, "I (A)" ("string"), w23, "R (Ohm)" ("string"), "\r\n") -> (w30:string)
      n12 = Build Path(base path="Folder", name or relative path=w19) -> (appended path=w18:path)
      n13 = flat-sequence {
        tunnel: w18 -> [w36]
        tunnel: w30 -> [w39]
        tunnel: [w39] -> w32
        tunnel: [w38] -> w27
        tunnel: [w37] -> w31
        tunnel: w32 -> [w46]
        tunnel: w31 -> [w45]
        frame #0 {
          n14 = Open/Create/Replace File(file path (use dialog)=w36, operation (0:open)=T1."create") -> (error out=w35:errorcluster)  [unwired: 4 in, 2 out]
          n15 = Unbundle By Name(w35) -> ("status"=w33:bool)
          n16 = case shown="True" w33 {
            tunnel: [FALSE ("Yes") w43] -> w38
            tunnel: [w40 w42] -> w37
            tunnel: w36 -> [w40 w42]
            frame False {
            }
            frame True {
              n17 = call "Message to User"() -> ("Yes"=w44:bool)  [unwired: 10 in, 1 out]
              n18 = Not(x=w44) -> (.not. x?=w43:bool)
            }
          }
        }
        frame #1 {
          n19 = call <vilib>:"Write Characters To File.vi"("append to file? (new file:F)"=TRUE, "character string"=w46, "file path (dialog if empty)"=w45) -> ()  [unwired: 2 in, 1 out]
          "File path" <- w45
        }
      }
      n20 = Stop(stop? (T)=w27) -> ()
    }
    frame #2 {
      n21 = Wait (ms)(milliseconds to wait=u32 1000) -> ()  [unwired: 1 out]
    }
    frame #3 {
      n22 = for {
        tunnel: "From" -> [w60] mode=indexing
        tunnel: "To" -> [w59] mode=indexing
        tunnel: "Step" -> [w58] mode=indexing
        shift-right: [w62] -> _
        shift-left: cluster{dbl, "Field Reading":dbl}[] [] -> [w63]
        shift-right: [w57] -> _
        shift-left: w51 -> [w64]
        shift-right: [w55] -> _
        shift-left: cluster{dbl, "Field Reading":dbl}[] [] -> [w56]
        n23 = call "Build_serie_EL.vi"("end value"=w59, "increment"=w58, "start value"=w60) -> ("output array"=w61:dbl[])
        n24 = for {
          tunnel: w61 -> [w70] mode=indexing
          shift-right: [w68] -> w62
          shift-left: w63 -> [w69]
          shift-right: [w67] -> w57
          shift-left: w64 -> [w71]
          shift-right: [w65] -> w55
          shift-left: w56 -> [w66]
          n25 = stacked-sequence {
            tunnel: w71 -> [w73 _ w83 _]
            tunnel: w69 -> [_ _ w88 _]
            tunnel: w70 -> [w72 _ _ _]
            tunnel: [_ _ w87 _] -> w68
            tunnel: [_ _ w82 _] -> w67
            tunnel: w66 -> [_ _ w79 _]
            tunnel: [_ _ w78 _] -> w65
            frame #0 {
              n26 = call "Configure Source (Level).vi"("VISA resource name"=w73, "Current Level (0 A)"=w72, "Source Measure Unit Channel (0: Channel A)"=0, "Level Type (1: Voltage)"=0) -> ()  [unwired: 10 in, 2 out]
            }
            frame #1 {
              n27 = Wait (ms)(milliseconds to wait="Wait (ms)") -> ()  [unwired: 1 out]
            }
            frame #2 {
              n28 = call-poly "Read Measurement.vi"("Wait Time (10 S)"=0, "Source Measure Unit Channel (0: Channel A)"=0, "VISA resource name"=w83) -> ("Last Voltage (V)"=w80:dbl, "Last Current (A)"=w84:dbl, "VISA resource name out"=w82:refnum<visa-resource-name>)  [unwired: 3 in, 3 out]
              "Current (A)" <- w84
              "Voltage (V)" <- w80
              n29 = Divide(x=w80, y=w84) -> (x/y=w77:dbl)
              "Resistance (ohm)" <- w77
              n30 = Bundle("Last Voltage (V)"=w80, "Last Current (A)"=w84) -> (w89:T2)  [unwired: 1 in]
              n31 = Build Array(w80, w84, w77) -> (→"data":dbl[])
              n32 = Build Array (concatenate)(w88, w89) -> (w87:T3)
              "I vs V" <- w87
              n33 = Bundle("Last Voltage (V)"=w80, w77) -> (w81:cluster{"Last Voltage (V)":dbl, dbl})  [unwired: 1 in]
              n34 = Build Array (concatenate)(w79, w81) -> (w78:T4)
              "R vs V" <- w78
            }
            frame #3 {
              n35 = local read "data"() -> (w91:dbl[])
              n36 = Array To Spreadsheet String(array=w91, 3:"%e" ("format string")) -> (spreadsheet string=w94:string)  [unwired: 1 in]
              n37 = local read "File path"() -> (w93:path)
              n38 = call <vilib>:"Write Characters To File.vi"("append to file? (new file:F)"=TRUE, "character string"=w94, "file path (dialog if empty)"=w93) -> ()  [unwired: 2 in, 1 out]
            }
          }
        }
      }
    }
    frame #4 {
      w99 = 0
      n39 = call "Configure Source (Level).vi"("VISA resource name"=w100, "Current Level (0 A)"=0.0, "Source Measure Unit Channel (0: Channel A)"=w99, "Level Type (1: Voltage)"=0) -> ("VISA resource name out"=w101:refnum<visa-resource-name>)  [unwired: 10 in, 1 out]
      n40 = call "Enable Source Output.vi"("Output Mode (0: Turn off)"=w99, "Source Measure Unit Channel (0: Channel A)"=w99, "VISA resource name"=w101) -> ("VISA resource name out"=w97:refnum<visa-resource-name>)  [unwired: 7 in, 1 out]
      n41 = call "Close.vi"("VISA resource name"=w97) -> ()  [unwired: 10 in, 1 out]
    }
  }
